vi "Run Test - Start Condition (SubVI).vi"(8 "error in (no error)":errorcluster, 9 "Time":dbl, 11 "Cluster in":T1 {"M Event" items=["Stop", "Running", "PID", "Up Limit", "Down Limit", "Load Limit"]; "Test Type" items=["Please Select", "Triaxial Shear", "Triaxial UU", "Shearbox", "Permeability", "Consolidation (Stepped Loading)/Swelling", "Saturation (Incremental)", "User Defined", "UCT", "Isotropic Consolidation", "Swelling Pressure"]; "Data"."Test Type" items=["Please Select", "Triaxial Shear", "Triaxial UU", "Shearbox", "Permeability", "Consolidation (Stepped Loading)/Swelling", "Saturation (Incremental)", "User Defined", "UCT", "Isotropic Consolidation", "Swelling Pressure"]}) -> (0 "error out":errorcluster, 2 "Delay":string, 3 "Cluster out":T1 {"M Event" items=["Stop", "Running", "PID", "Up Limit", "Down Limit", "Load Limit"]; "Test Type" items=["Please Select", "Triaxial Shear", "Triaxial UU", "Shearbox", "Permeability", "Consolidation (Stepped Loading)/Swelling", "Saturation (Incremental)", "User Defined", "UCT", "Isotropic Consolidation", "Swelling Pressure"]; "Data"."Test Type" items=["Please Select", "Triaxial Shear", "Triaxial UU", "Shearbox", "Permeability", "Consolidation (Stepped Loading)/Swelling", "Saturation (Incremental)", "User Defined", "UCT", "Isotropic Consolidation", "Swelling Pressure"]}, 5 "Enum":T10)   [LabVIEW 2019]
uses:
  Controls/RunTest - State.ctl
  Controls/RunTest - Data Structure.ctl
  Controls/Test Panel - Data Structure.ctl
  Controls/Station - Test Type.ctl
  <vilib>/Utility/miscctls.llb/LVRowAndColumnTypeDef.ctl
  Controls/RunTest - Calculate Data.ctl
  <vilib>/httpClient/ClientHandle.ctl
  Controls/RunTest - Start Condition.ctl
  Controls/RunTest - Stop Condition.ctl
  Controls/UDP - Event.ctl
  Controls/UDP - Command.ctl
  <vilib>/httpClient/LabVIEWHTTPClient.lvlib
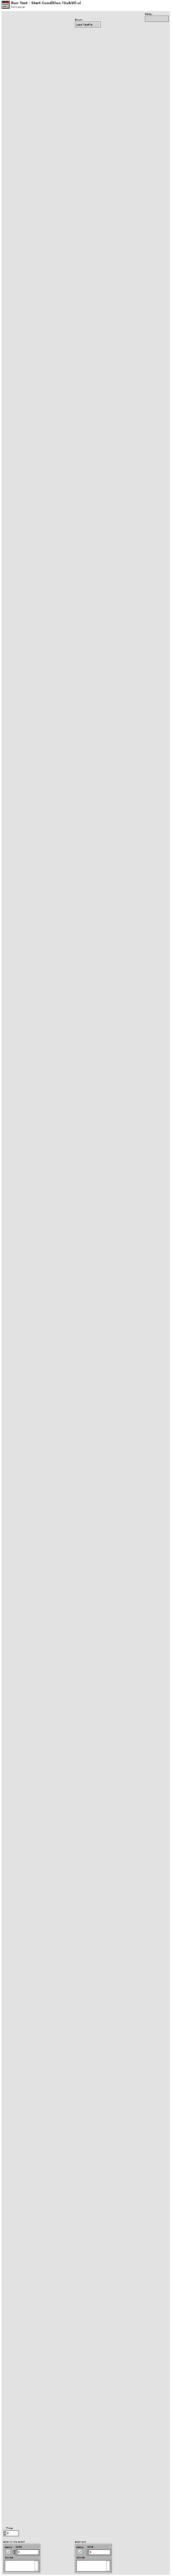
[diagram p1: front panel]
types:
  T1 = typedef "RunTest - Data Structure.ctl" = cluster{"Test Plan":string[], "PlanRow":i32, "Device Name":string[], "Timeout":i32, "Start?":bool, "Pause?":bool, "IP Address":string[], "LogRow":i32, "Logtype":u16, "Log Elapse":sgl, "Data":T2, "Stop log?":bool, "tdms":refnum<k34>, "Sensor Data":sgl[], "Start time":timestamp, "Prev Log Elapse":u32, "Plot":u16, "X-Axis":u16[], "Y-Axis":u16[], "XY":cluster{"X":dbl, "Y":dbl}[][], "End Stage?":bool, "1run":bool, "Condition":u16[], "Start Con":bool, "Log Con":bool, "Stop Con":bool, "Start Elapse":dbl, "Start Load":dbl, "Motor":i32, "StartRow":i32, "number log":i32, "Dir":bool, "Start time test":timestamp, "Auto":bool, "Check return?":bool, "Inv":cluster{"M":i32[], "Bool":bool[]}, "tdms temp":refnum<k34>, "Zero?":bool, "Plot Timer":dbl, "1st Run":bool, "TDMS Path":path, "MaxLoad":dbl, "Log Timer":sgl[], "Test Type":T3, "Log Sensor":string[], "Save?":bool, "1st Log":bool, "Y-Axis 2":u16[], "On Y-Axis 2":bool, "Decimal":u8[], "Init":cluster{"PWP TS":sgl, "Load TS":sgl, "Volume TS":sgl, "Disp TS":sgl, "CP":sgl, "Vol In":sgl, "Vol Out":sgl, "Load UCT":sgl, "Disp UCT":sgl, "PWP Sat":sgl, "CP Sat":sgl, "Volume IsoCons":sgl, "PWP IsoCons":sgl, "PWP TUU":sgl, "Load TUU":sgl, "Volume TUU":sgl, "Disp TUU":sgl, "Load Cons":sgl, "Disp Cons":sgl, "Volume Sat":sgl, "Vertical Load SB":sgl, "Vertical Disp SB":sgl, "H Disp SB":sgl, "H Load SB":sgl}, "Calc":T5, "Device Index":i32[], "Channel Index":i32[], "http ref":T6, "fileid":string, "Step Cons":cluster{"V Stress":sgl, "H Settlement":sgl}, "RunTest":bool, "Graph Last":i32, "Init?":bool, "Datalog":bool[], "Start":T7, "Stop":T8, "Running?":bool, "StartTime":dbl, "Log Prev Time":dbl, "KeyName":string[], "Test RunTime":dbl, "Log Prev Axial":dbl, "M Event":T9[], "Last Log":bool, "popup":bool, "PreStart UU":bool, "PreStart Sat":bool}
  T2 = typedef "Test Panel - Data Structure.ctl" = cluster{"Station":string, "Sample ID":string, "Job No":string, "Job Description":string, "Filename":string, "Test Type":T3, "Speciment No":string, "Depth":string, "Height":string, "Diameter/Length":string, "Weight":string, "Test Parameter":string, "Station[]":string[], "Edit Pos":T4, "Edit Pos Prev":T4, "Area":string, "Path":string}
  T3 = typedef "Station - Test Type.ctl" = u16
  T4 = typedef "LVRowAndColumnTypeDef.ctl" = cluster{"Row":i32, "Column":i32}
  T5 = typedef "RunTest - Calculate Data.ctl" = cluster{"TS":cluster{"Change PWP":sgl, "Change Vol":sgl, "Axial Load":sgl, "CiL":sgl, "Deviator":sgl, "Axial Strain":sgl, "MaxDeviator":sgl}, "TUU":cluster{"Change PWP":sgl, "Axial Load":sgl, "CiL":sgl, "Deviator":sgl, "Axial Strain":sgl, "MaxDeviator":sgl}, "Sat":cluster{"B Value":sgl, "PWP Diss":sgl, "CPP":sgl, "CV":sgl}, "Per":cluster{"Change Vol In":sgl, "Change Vol Out":sgl, "Mean Vol":sgl, "Gradient Pressure":sgl, "Outlet Flow":sgl, "Inlet Flow":sgl, "I X1":sgl, "I X2":sgl, "I Y1":sgl, "I Y2":sgl, "O X1":sgl, "O X2":sgl, "O Y1":sgl, "O Y2":sgl}, "Step Cons":cluster{"V Stress":sgl, "H Settlement":sgl, "Total H Settle":sgl, "Prev Total H":sgl}, "UCT":cluster{"ALC":sgl, "H Change":sgl, "Deviator":sgl, "Axial Strain":sgl, "V Stress":sgl, "MaxDeviator":sgl}, "ISO Cons":cluster{"CPP":sgl, "PWP Diss":sgl, "CV":sgl}, "SB":cluster{"Speci LenC":sgl, "Shear Strain":sgl, "H LC":sgl, "Normal Stress":sgl, "Shear Stress":sgl, "MaxShear":sgl}}
  T6 = typedef "LabVIEWHTTPClient.lvlib/ClientHandle.ctl" = refnum<k1>
  T7 = typedef "RunTest - Start Condition.ctl" = cluster{"Cons":cluster{"VS":dbl, "Delay":bool, "No Delay":dbl}, "Sat":cluster{"CP":dbl, "BP":dbl, "StartBP":bool, "Target CP":bool, "Target BP":bool}, "Iso":cluster{"BP":dbl}, "TS":cluster{"SS":dbl, "Engage":bool, "ES":dbl, "LC":dbl, "PreStart":bool, "Trig SS":bool, "Drain":dbl}, "TUU":cluster{"SS":dbl, "Engage":bool, "ES":dbl, "LC":dbl, "PreStart":bool, "Trig SS":bool, "CP":dbl, "Delay Value":dbl, "Delay":bool, "CP PID":bool}, "UCT":cluster{"SS":dbl, "Engage":bool, "ES":dbl, "LC":dbl, "PreStart":bool, "Trig SS":bool}, "Enable?":bool, "SB":cluster{"SS":dbl, "Engage":bool, "ES":dbl, "LC":dbl, "PreStart":bool, "Trig SS":bool, "VS":dbl, "Delay Value":dbl, "Delay":bool, "VS PID":bool}, "Perm":cluster{"DP":dbl}}
  T8 = typedef "RunTest - Stop Condition.ctl" = cluster{"Cons":cluster{"Select":i32, "Disp":dbl, "Time":dbl, "Time2":dbl, "Disp 2":dbl, "Time Cond":dbl, "Last Disp":dbl, "Swell":bool}, "Sat":cluster{"Select":i32, "PP":dbl, "Time":dbl, "VC":dbl, "Time2":dbl, "Time Cond":dbl, "Last PP":dbl, ".B":bool, "B":dbl, "Last Vc":dbl, "Time Cond 2":dbl, "Time3":dbl, "Time Cond 3":dbl}, "Iso":cluster{"PP":dbl, "Time":dbl, "VC":dbl, "Time2":dbl, "Time Cond":dbl, "Last Vc":dbl, ".PP":bool, "Time Cond 2":dbl, "Select":i32}, "TS":cluster{"Axial":dbl, ".MaxDev":bool, "MaxDev Value":dbl, "Return":bool, "Reset":bool, "Prev Time":dbl, "PostStop Run":bool, "CP Stop":bool, "BP Stop":bool, "PostStop Trig":bool, "Reset Value":dbl, "BPTrig":bool, "CPTrig":bool, "VLCTrig":bool}, "TUU":cluster{"Axial":dbl, ".MaxDev":bool, "MaxDev Value":dbl, "Return":bool, "Reset":bool, "Prev Time":dbl, "PostStop Run":bool, "CP Stop":bool, "BP Stop":bool, "PostStop Trig":bool, "Reset Value":dbl, "BPTrig":bool, "CPTrig":bool, "VLCTrig":bool}, "UCT":cluster{"Axial":dbl, ".MaxDev":bool, "MaxDev Value":dbl, "Return":bool, "Reset":bool, "Prev Time":dbl, "PostStop Run":bool, "CP Stop":bool, "BP Stop":bool, "PostStop Trig":bool}, "Enable?":bool, "SB":cluster{"Shear":dbl, ".MaxShear":bool, "MaxShear Value":dbl, "Return":bool, "Reset":bool, "Prev Time":dbl, "PostStop Run":bool, "CP Stop":bool, "BP Stop":bool, "PostStop Trig":bool, "Reset Value":dbl, "BPTrig":bool, "CPTrig":bool, "VLCTrig":bool}, "Perm":cluster{"Max Time":bool, "Reset":bool, "PostStop Run":bool, "Ratio":bool, "Reset Value":dbl, "Time":dbl, "RatioTime":dbl, "RatioMore":dbl, "RatioLess":dbl, "Time Cond":dbl, "Time Cond 2":dbl, "Prev IF":dbl, "Prev OF":dbl, "PostStop Trig":bool, "BP Trig":bool, "DP Stop":bool, "BP Stop":bool, "CP Stop":bool, "CP Trig":bool}, "SP":cluster{".Max Time":bool, ".Time":bool, "Time":dbl, "MaxTime":dbl, "Time Cond":dbl, "Max Time Cond":dbl, "Stress":dbl}}
  T9 = typedef "UDP - Event.ctl" = u16
  T10 = typedef "RunTest - State.ctl" = enum16{"Load Testfile", "Notifier", "Init", "Idle", "Load", "Read DB", "Run", "Pause", "Stop", "Check Start", "Check Stop", "Check Post Stop", "Check Log", "EndStage", "Data View", "Display", "Graph", "Graph Old", "Close", "Stop PID", "Check Limit", "Auto", "Up", "Log", "Zero", "Machine Control", "Save Report"}
  T11 = enum32{"Please Select", "Triaxial Shear", "Triaxial UU", "Shearbox", "Permeability", "Consolidation", "Saturation", "User Defined", "UCT", "Iso Consolidation"}
  T12 = cluster{"Target Load":sgl, "Target Disp":sgl, "Rate":sgl, "Speed":sgl}
  T13 = enum16{"None", "Run Target", "Run Ramp", "Run Disp"}
  T14 = typedef "UDP - Command.ctl" = enum16{"Stop", "Jog Up", "Jog Down", "Ramp Up", "Ramp Down", "PID Target", "PID Ramp", "Disp Run", "Read Ch Data", "Zero Channel", "Zero Disp", "Read Sensor", "Write Sensor", "Read ADC", "Write ADC", "Read PID", "Write PID", "Read Test", "Write Test", "Read System", "Write System", "Read Datalog", "Read Datalog Sensor"}
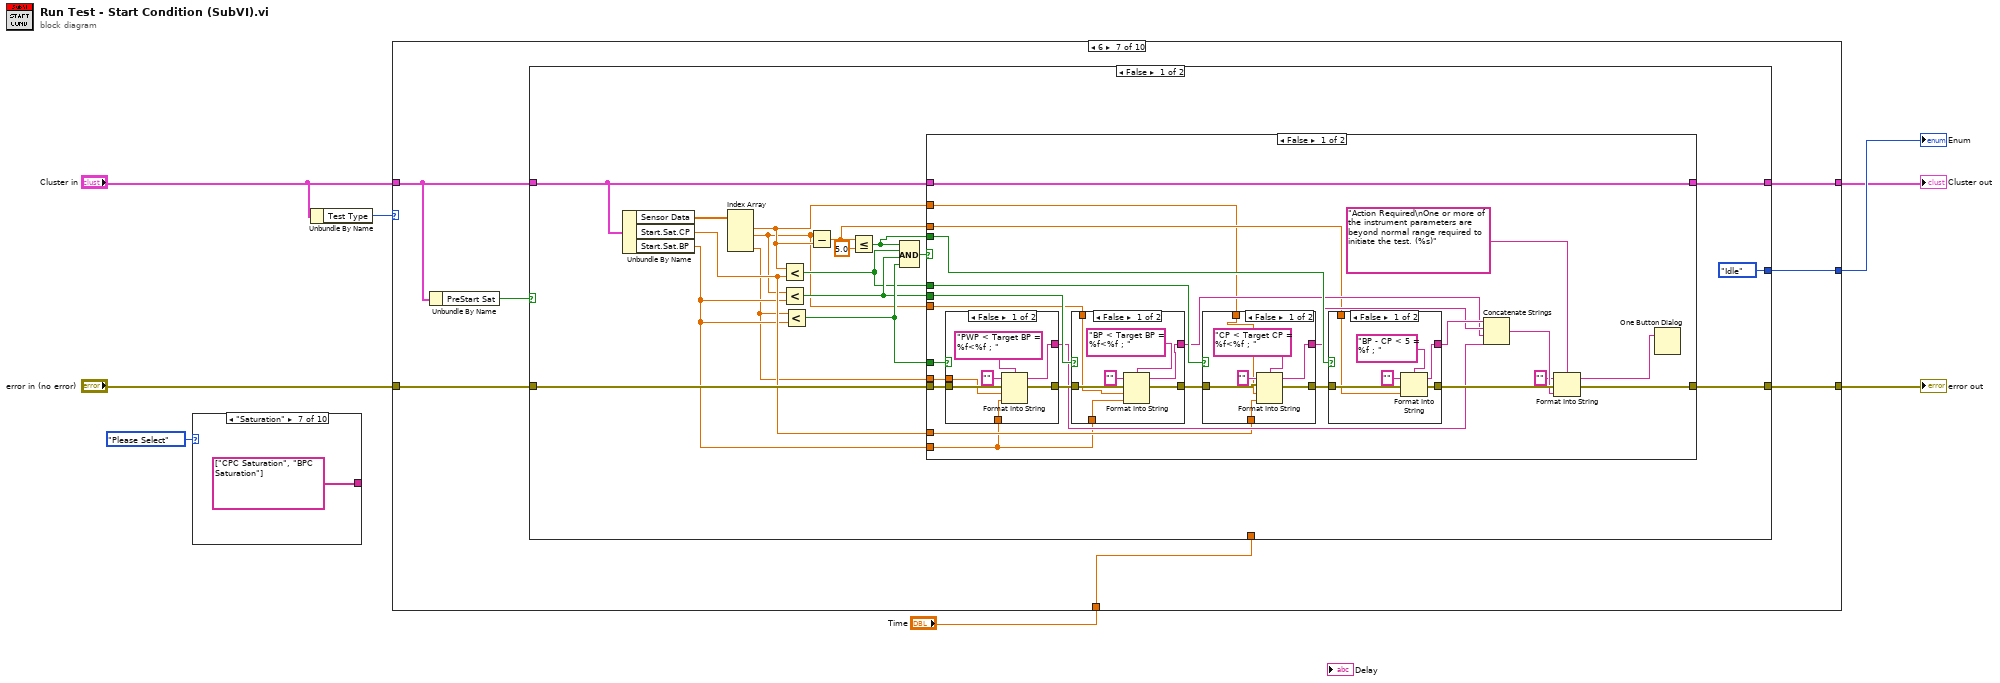
[diagram p0: block diagram]
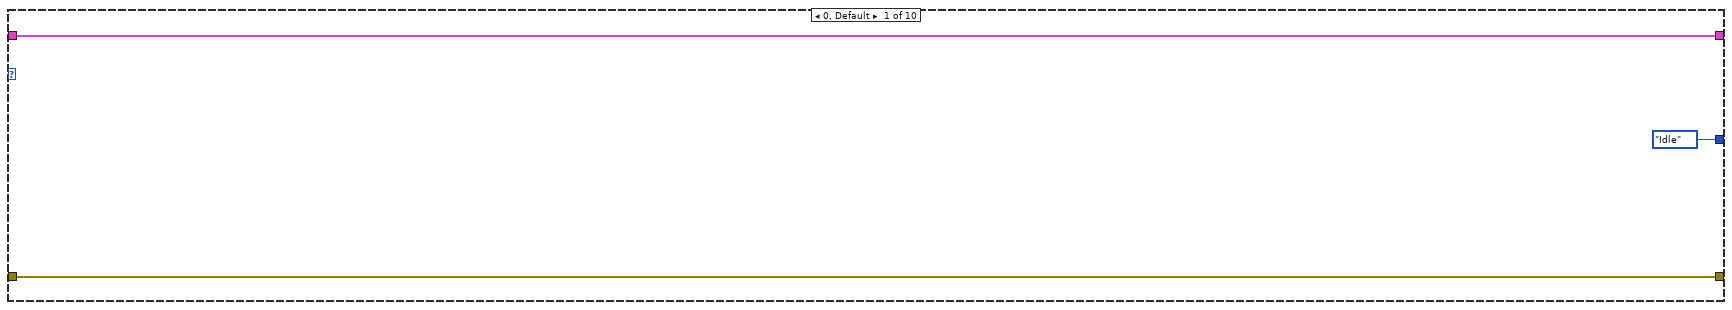
[diagram p2: hidden frame]
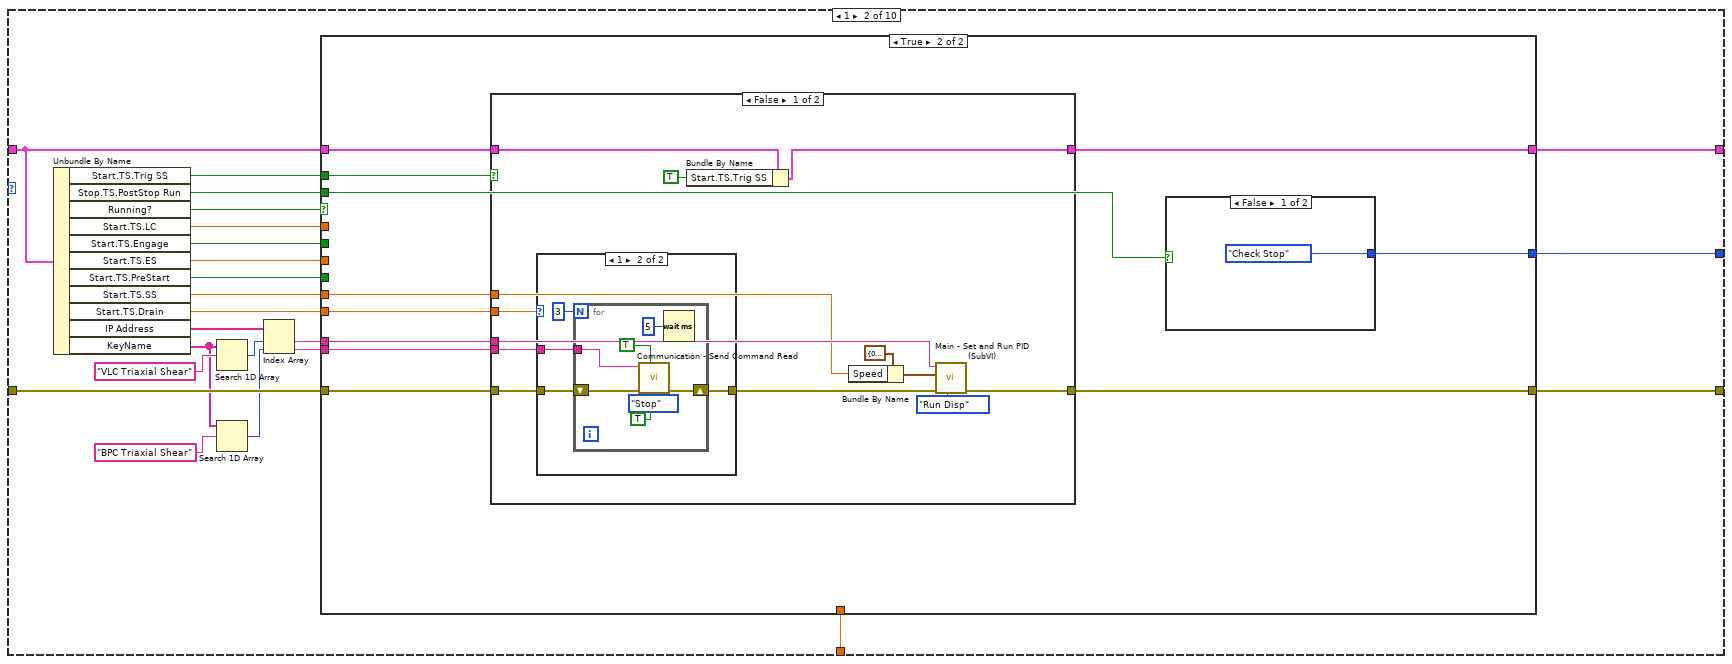
[diagram p3: hidden frame]
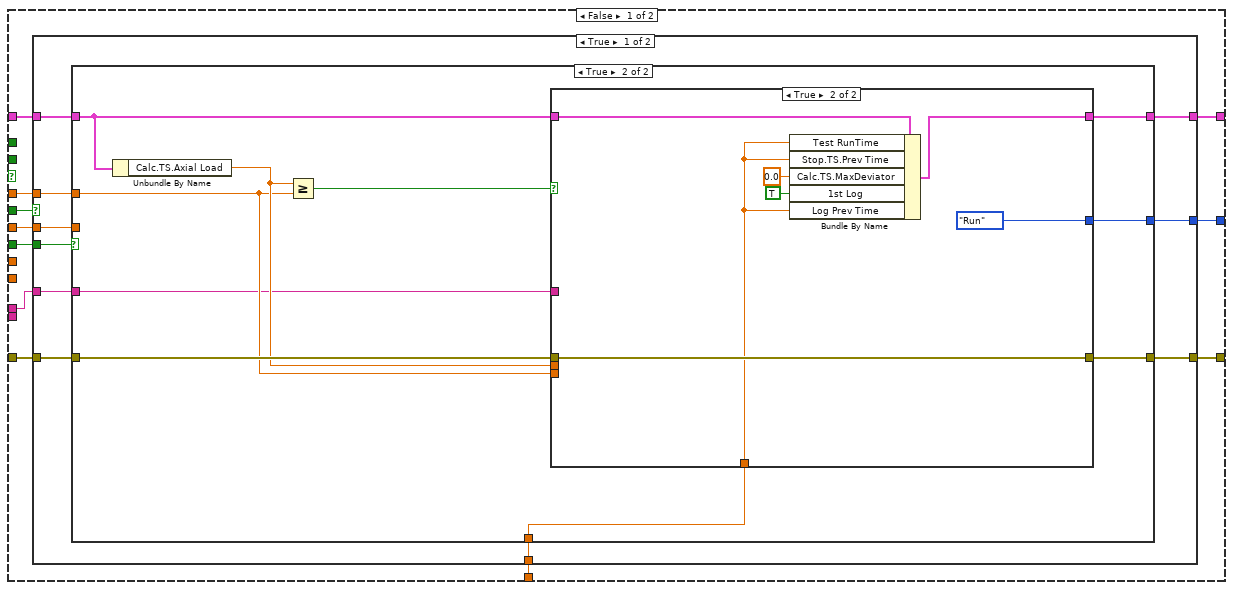
[diagram p4: hidden frame]
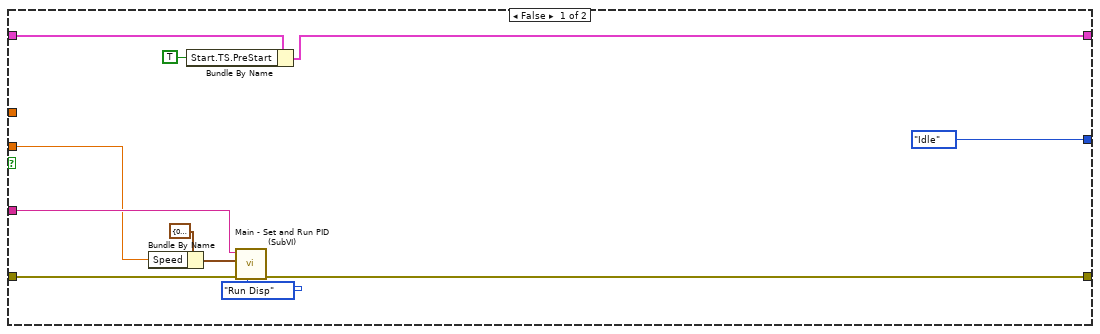
[diagram p5: hidden frame]
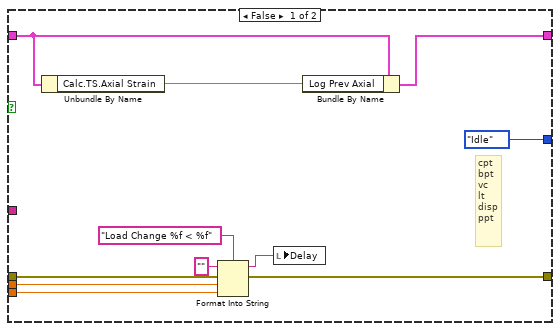
[diagram p6: hidden frame]
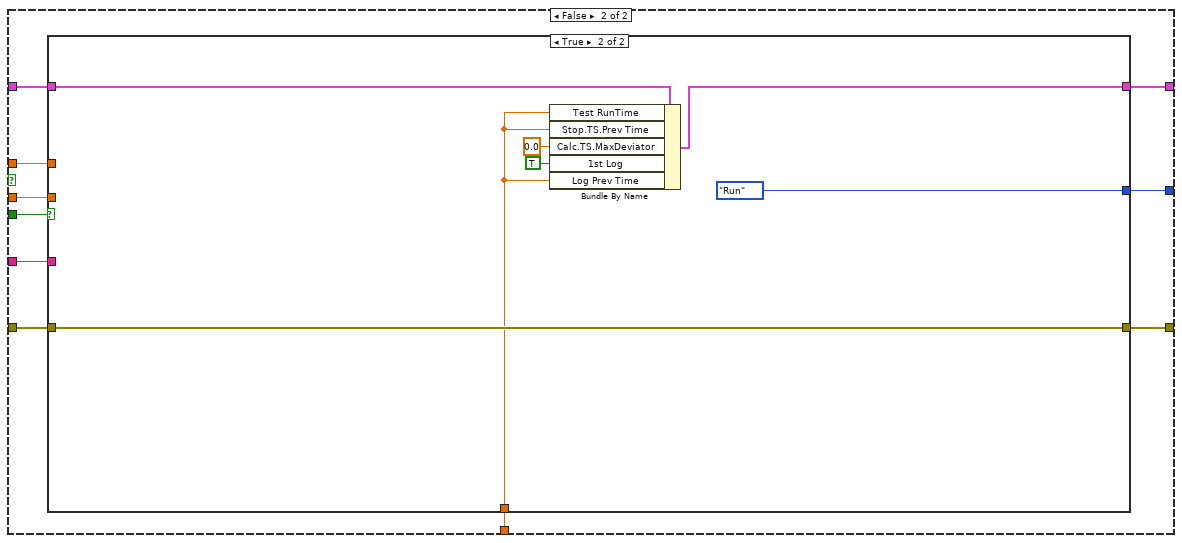
[diagram p7: hidden frame]
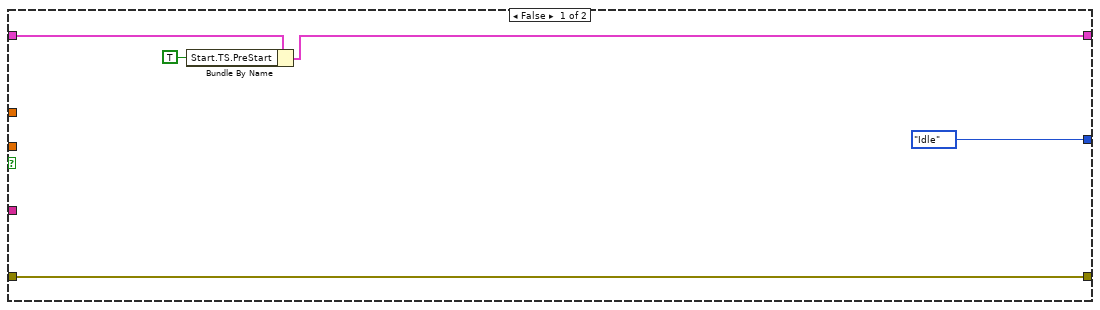
[diagram p8: hidden frame]
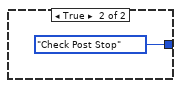
[diagram p11: hidden frame]
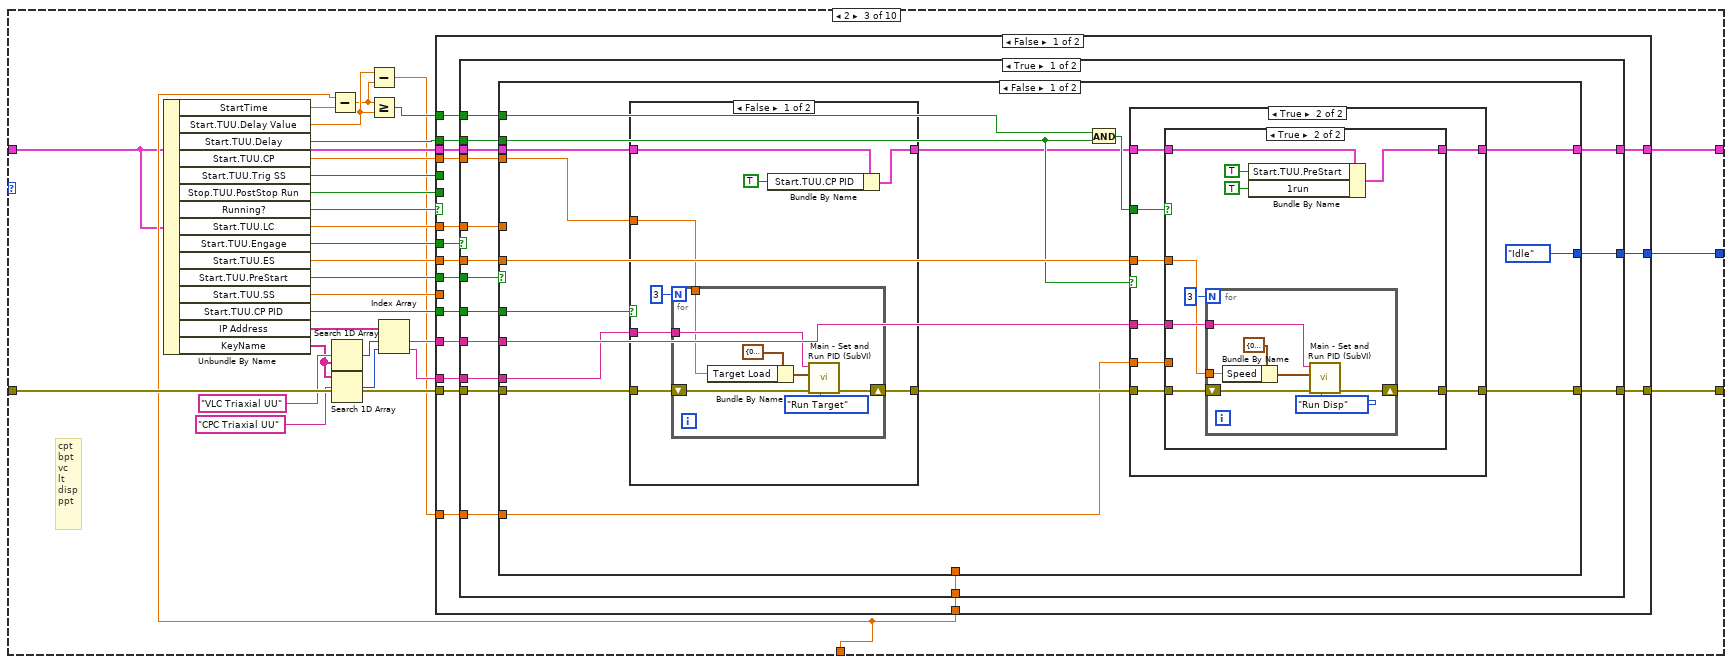
[diagram p12: hidden frame]
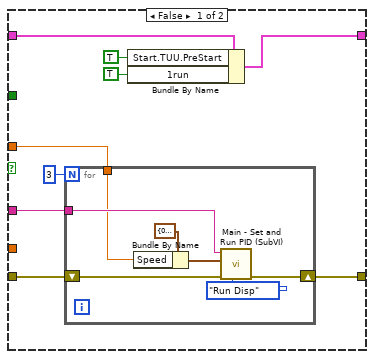
[diagram p13: hidden frame]
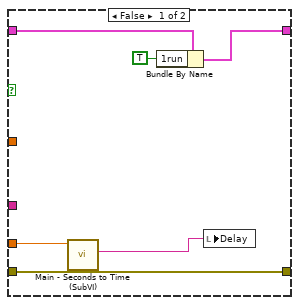
[diagram p14: hidden frame]
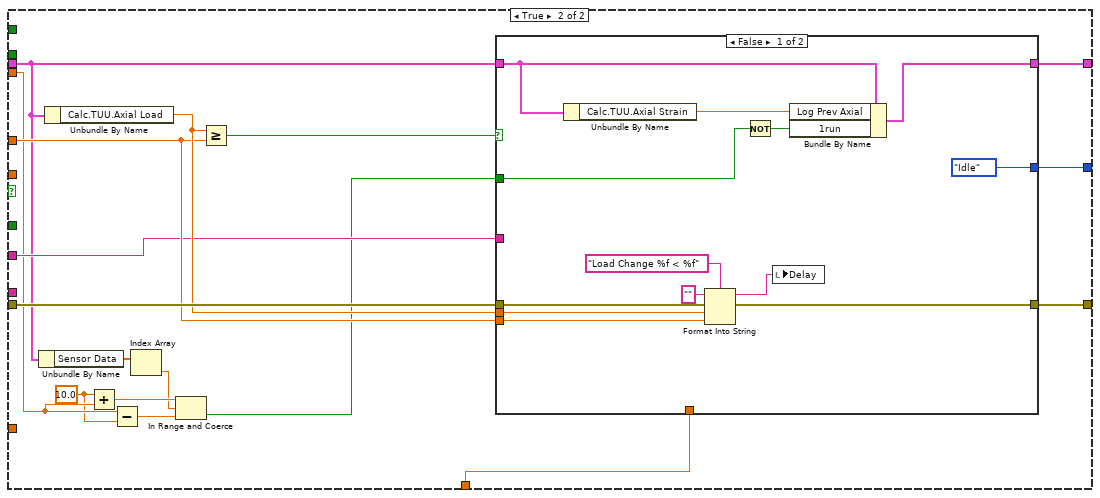
[diagram p16: hidden frame]
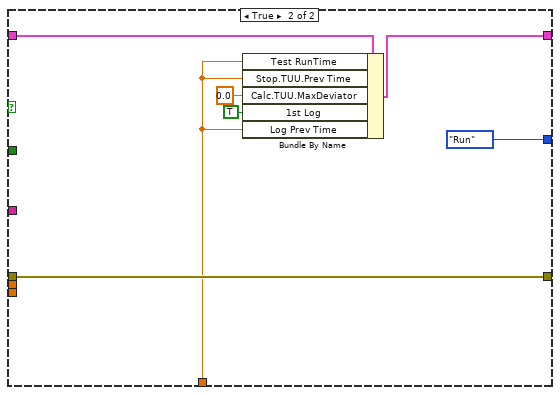
[diagram p17: hidden frame]
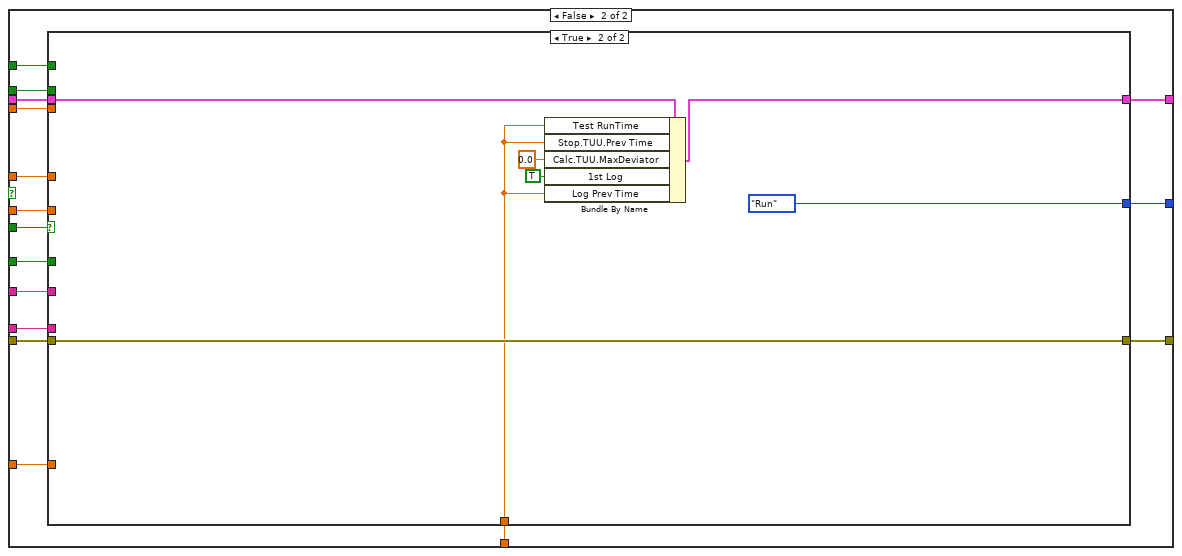
[diagram p18: hidden frame]
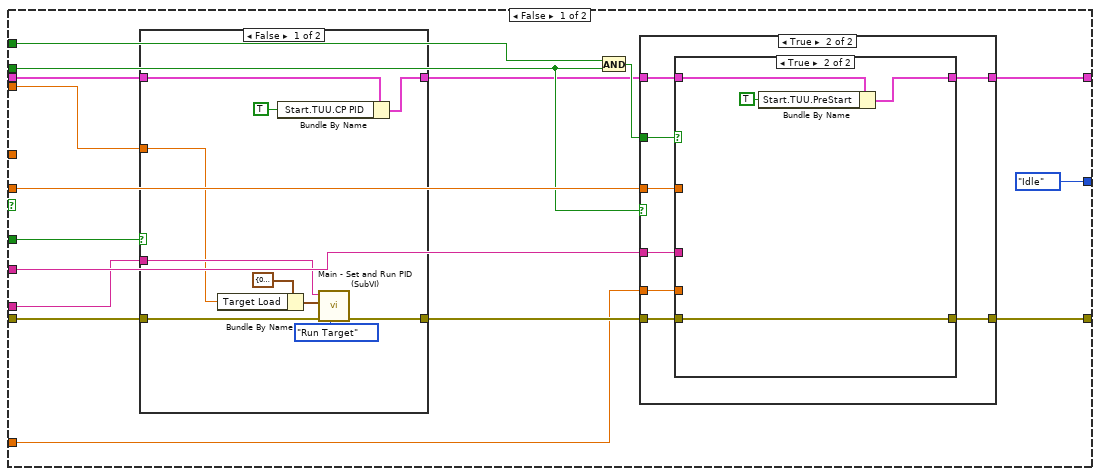
[diagram p19: hidden frame]
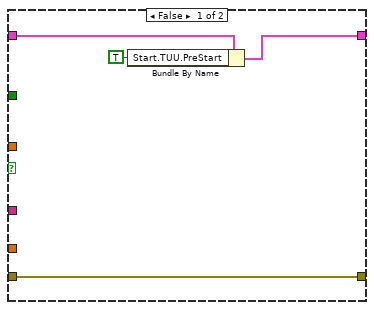
[diagram p20: hidden frame]
diagram:
  n1 = case shown="\"Saturation\"" T11."Please Select" ("Sub Tab") {
    tunnel: [string[] [] string[] ["CPC Triaxial Shear", "BPC Triaxial Shear", "VLC Triaxial Shear"] string[] ["CPC Triaxial UU", "VLC Triaxial UU"] string[] ["VLC Shearbox", "HLC Shearbox"] string[] ["CPC Permeability", "BPC Permeability", "BPC2 Permeability"] string[] ["VLC Consolidation"] string[] ["CPC Saturation", "BPC Saturation"] string[] ["CPC User Defined", "BPC User Defined", "BPC2 User Defined", "VLC User Defined", "HLC User Defined"] string[] ["VLC UCT"] string[] ["CPC Iso", "BPC Iso"]] -> _
    frame "Please Select", Default {
    }
    frame "Triaxial Shear" {
    }
    frame "Triaxial UU" {
    }
    frame "Shearbox" {
    }
    frame "Permeability" {
    }
    frame "Consolidation" {
    }
    frame "Saturation" {
    }
    frame "User Defined" {
    }
    frame "UCT" {
    }
    frame "Iso Consolidation" {
    }
  }
  n2 = Unbundle By Name("Cluster in") -> ("Test Type"=w1:T3)
  n3 = case shown="6" w1 {
    tunnel: [w21 w39 w195 w464 w708 w773 w953 w1243 w1359 w1426] -> w3
    tunnel: "Cluster in" -> [w21 w40 w191 w465 w707 w772 w951 w1244 w1358 w1425]
    tunnel: [w20 w38 w194 w463 w714 w779 w956 w1242 w1364 w1430] -> w5
    tunnel: "error in (no error)" -> [w20 w43 w196 w468 w713 w778 w955 w1247 w1363 w1429]
    tunnel: [RunTest_-_State."Idle" w36 w193 w461 w712 w777 w954 w1240 w1362 w1428] -> w6
    tunnel: "Time" -> [_ w27 w192 w440 w702 w765 w952 w1230 w1354 w1424]
    frame 0, Default {
    }
    frame 1 {
      n4 = Unbundle By Name(w40) -> ("Start.TS.Trig SS"=w28:bool, "Stop.TS.PostStop Run"=w29:bool, "Running?"=w31:bool, "Start.TS.LC"=w37:dbl, "Start.TS.Engage"=w41:bool, "Start.TS.ES"=w42:dbl, "Start.TS.PreStart"=w44:bool, "Start.TS.SS"=w30:dbl, "Start.TS.Drain"=w22:dbl, "IP Address"=w34:string[], "KeyName"=w25:string[])
      n5 = Search 1D Array(1D array=w25, element="VLC Triaxial Shear" ("String")) -> (index of element=w35:i32)  [unwired: 1 in]
      n6 = Search 1D Array(1D array=w25, element="BPC Triaxial Shear" ("String")) -> (index of element=w24:i32)  [unwired: 1 in]
      n7 = Index Array(array=w34, index #1=w35, index #2=w24) -> (element #1=w32:string, element #2=w23:string)
      n8 = case shown="True" w31 {
        tunnel: w44 -> [w55 _]
        tunnel: w43 -> [w54 w134]
        tunnel: w42 -> [w53 _]
        tunnel: w41 -> [w52 _]
        tunnel: w40 -> [w51 w129]
        tunnel: [w50 w130] -> w39
        tunnel: [w49 w135] -> w38
        tunnel: w37 -> [w48 _]
        tunnel: [w47 w137] -> w36
        tunnel: w32 -> [w46 w133]
        tunnel: w30 -> [_ w132]
        tunnel: w29 -> [_ w136]
        tunnel: w28 -> [_ w131]
        tunnel: w27 -> [w45 _]
        tunnel: w23 -> [_ w128]
        tunnel: w22 -> [_ w127]
        frame False {
          n9 = case shown="True" w52 {
            tunnel: w55 -> [w65 w114]
            tunnel: w54 -> [w64 w113]
            tunnel: w53 -> [w63 w112]
            tunnel: [w62 w111] -> w49
            tunnel: w51 -> [w61 w110]
            tunnel: [w60 w109] -> w50
            tunnel: w48 -> [w59 w108]
            tunnel: [w58 w107] -> w47
            tunnel: w46 -> [w57 w106]
            tunnel: w45 -> [w56 w105]
            frame True {
              n10 = case shown="True" w65 {
                tunnel: w64 -> [w73 w84]
                tunnel: [w72 w85] -> w62
                tunnel: w63 -> [w66 _]
                tunnel: w61 -> [w71 w78]
                tunnel: [w69 w79] -> w60
                tunnel: w59 -> [_ w82]
                tunnel: [RunTest_-_State."Idle" w86] -> w58
                tunnel: w57 -> [w68 w80]
                tunnel: w56 -> [_ w77]
                frame False {
                  n11 = Bundle By Name(cluster=T12 {"Target Load"=0.0, "Target Disp"=0.0, "Rate"=0.0, "Speed"=0.0} ("Test"), "Speed"=w66) -> (w76:T12)
                  n12 = Bundle By Name(cluster=w71, "Start.TS.PreStart"=TRUE) -> (w69:T1)
                  n13 = call "Main - Set and Run PID (SubVI).vi"("Action"=T13."Run Disp", "error in (no error)"=w73, "Test"=w76, "IP Address"=w68) -> ("error out"=w72:errorcluster)  [unwired: 7 in]
                }
                frame True {
                  n14 = Unbundle By Name(w78) -> ("Calc.TS.Axial Load"=w83:sgl)
                  n15 = Greater Or Equal?(x=w83, y=w82) -> (x >= y?=w81:bool)
                  n16 = case shown="True" w81 {
                    tunnel: [RunTest_-_State."Idle" RunTest_-_State."Run"] -> w86
                    tunnel: [w97 w100] -> w85
                    tunnel: w84 -> [w96 w100]
                    tunnel: w83 -> [w94 _]
                    tunnel: w82 -> [w93 _]
                    tunnel: w80 -> [_ _]
                    tunnel: [w90 w103] -> w79
                    tunnel: w78 -> [w89 w102]
                    tunnel: w77 -> [_ w98]
                    frame False {
                      # "cpt\nbpt\nvc\nlt\ndisp\nppt"
                      n17 = Unbundle By Name(w89) -> ("Calc.TS.Axial Strain"=w88:sgl)
                      n18 = Format Into String(format string="Load Change %f < %f" ("Delay"), initial string="", error in=w96, w94, w93) -> (resulting string=w87:string, error out=w97:errorcluster)
                      n19 = local write "Delay"(w87) -> ()
                      n20 = Bundle By Name(cluster=w89, "Log Prev Axial"=w88) -> (w90:T1)
                    }
                    frame True {
                      n21 = Bundle By Name(cluster=w102, "Test RunTime"=w98, "Stop.TS.Prev Time"=w98, "Calc.TS.MaxDeviator"=sgl 0.0, "1st Log"=TRUE, "Log Prev Time"=w98) -> (w103:T1)
                    }
                  }
                }
              }
            }
            frame False {
              n22 = case shown="True" w114 {
                tunnel: w113 -> [w119 w125]
                tunnel: [w119 w125] -> w111
                tunnel: w112 -> [_ _]
                tunnel: w110 -> [w118 w123]
                tunnel: [w116 w124] -> w109
                tunnel: w108 -> [_ _]
                tunnel: [RunTest_-_State."Idle" RunTest_-_State."Run"] -> w107
                tunnel: w106 -> [_ _]
                tunnel: w105 -> [_ w122]
                frame False {
                  n23 = Bundle By Name(cluster=w118, "Start.TS.PreStart"=TRUE) -> (w116:T1)
                }
                frame True {
                  n24 = Bundle By Name(cluster=w123, "Test RunTime"=w122, "Stop.TS.Prev Time"=w122, "Calc.TS.MaxDeviator"=sgl 0.0, "1st Log"=TRUE, "Log Prev Time"=w122) -> (w124:T1)
                }
              }
            }
          }
        }
        frame True {
          n25 = case shown="False" w131 {
            tunnel: [w148 w163] -> w135
            tunnel: w134 -> [w141 w163]
            tunnel: w133 -> [w147 _]
            tunnel: w132 -> [w143 _]
            tunnel: [w146 w164] -> w130
            tunnel: w129 -> [w145 w164]
            tunnel: w128 -> [w140 _]
            tunnel: w127 -> [w142 _]
            frame False {
              n26 = case shown="1" w142 {
                tunnel: w141 -> [w151 w155]
                tunnel: w140 -> [_ w153]
                tunnel: [w151 w154] -> w139
                frame 0, Default {
                }
                frame 1 {
                  n27 = for {
                    N: 3 -> [_]
                    tunnel: w153 -> [w157]
                    shift-right: [w158] -> w154
                    shift-left: w155 -> [w159]
                    n28 = call "Communication - Send Command Read.vi"("Fron?"=TRUE, "Bypass?"=TRUE, "error in (no error)"=w159, "Action"=UDP_-_Command."Stop", "Device IP Address"=w157) -> ("error out"=w158:errorcluster)  [unwired: 6 in]
                    n29 = Wait (ms)(milliseconds to wait=u32 5) -> ()  [unwired: 1 out]
                  }
                }
              }
              n30 = Bundle By Name(cluster=w145, "Start.TS.Trig SS"=TRUE) -> (w146:T1)
              n31 = Bundle By Name(cluster=T12 {"Target Load"=0.0, "Target Disp"=0.0, "Rate"=0.0, "Speed"=0.0} ("Test"), "Speed"=w143) -> (w150:T12)
              n32 = call "Main - Set and Run PID (SubVI).vi"("Action"=T13."Run Disp", "error in (no error)"=w139, "Test"=w150, "IP Address"=w147) -> ("error out"=w148:errorcluster)  [unwired: 7 in]
            }
            frame True {
            }
          }
          n33 = case shown="False" w136 {
            tunnel: [RunTest_-_State."Check Stop" RunTest_-_State."Check Post Stop"] -> w137
            frame False {
            }
            frame True {
            }
          }
        }
      }
    }
    frame 2 {
      # "cpt\nbpt\nvc\nlt\ndisp\nppt"
      n34 = Unbundle By Name(w191) -> ("StartTime"=w172:dbl, "Start.TUU.Delay Value"=w169:dbl, "Start.TUU.Delay"=w173:bool, "Start.TUU.CP"=w178:dbl, "Start.TUU.Trig SS"=w179:bool, "Stop.TUU.PostStop Run"=w180:bool, "Running?"=w182:bool, "Start.TUU.LC"=w187:dbl, "Start.TUU.Engage"=w188:bool, "Start.TUU.ES"=w189:dbl, "Start.TUU.PreStart"=w190:bool, "Start.TUU.SS"=w181:dbl, "Start.TUU.CP PID"=w170:bool, "IP Address"=w185:string[], "KeyName"=w177:string[])
      n35 = Subtract(x=w192, y=w172) -> (x-y=w168:dbl)
      n36 = Search 1D Array(1D array=w177, element="VLC Triaxial UU" ("String")) -> (index of element=w186:i32)  [unwired: 1 in]
      n37 = Search 1D Array(1D array=w177, element="CPC Triaxial UU" ("String")) -> (index of element=w175:i32)  [unwired: 1 in]
      n38 = Subtract(x=w169, y=w168) -> (x-y=w167:dbl)
      n39 = Greater Or Equal?(x=w168, y=w169) -> (x >= y?=w171:bool)
      n40 = Index Array(array=w185, index #1=w186, index #2=w175) -> (element #1=w183:string, element #2=w174:string)
      n41 = case shown="False" w182 {
        tunnel: w190 -> [w213 _]
        tunnel: w196 -> [w212 w422]
        tunnel: w189 -> [w211 _]
        tunnel: w188 -> [w210 _]
        tunnel: w191 -> [w209 w417]
        tunnel: [w208 w418] -> w195
        tunnel: [w207 w423] -> w194
        tunnel: w187 -> [w206 _]
        tunnel: [w205 w425] -> w193
        tunnel: w183 -> [w204 w421]
        tunnel: w181 -> [_ w420]
        tunnel: w180 -> [_ w424]
        tunnel: w179 -> [_ w419]
        tunnel: w178 -> [w203 _]
        tunnel: w174 -> [w202 _]
        tunnel: w173 -> [w201 _]
        tunnel: w171 -> [w200 _]
        tunnel: w170 -> [w199 _]
        tunnel: w167 -> [w198 _]
        tunnel: w192 -> [w197 _]
        frame False {
          n42 = case shown="True" w210 {
            tunnel: w213 -> [w229 w361]
            tunnel: w212 -> [w228 w360]
            tunnel: w211 -> [w227 w359]
            tunnel: [w226 w358] -> w207
            tunnel: w209 -> [w225 w357]
            tunnel: [w224 w356] -> w208
            tunnel: w206 -> [w223 w355]
            tunnel: [w222 w354] -> w205
            tunnel: w204 -> [w221 w353]
            tunnel: w203 -> [w220 w352]
            tunnel: w202 -> [w219 w351]
            tunnel: w201 -> [w218 w350]
            tunnel: w200 -> [w217 w349]
            tunnel: w199 -> [w216 w348]
            tunnel: w198 -> [w215 w347]
            tunnel: w197 -> [w214 w346]
            frame True {
              n43 = case shown="False" w229 {
                tunnel: w228 -> [w237 w323]
                tunnel: [w239 w324] -> w226
                tunnel: w227 -> [w242 _]
                tunnel: w225 -> [w232 w313]
                tunnel: [w245 w319] -> w224
                tunnel: w223 -> [_ w321]
                tunnel: [RunTest_-_State."Idle" w325] -> w222
                tunnel: w221 -> [w244 w320]
                tunnel: w220 -> [w240 w311]
                tunnel: w219 -> [w241 _]
                tunnel: w218 -> [w235 _]
                tunnel: w217 -> [w236 _]
                tunnel: w216 -> [w233 _]
                tunnel: w215 -> [w231 _]
                tunnel: w214 -> [_ w318]
                frame False {
                  n44 = case shown="False" w233 {
                    tunnel: w241 -> [w299 _]
                    tunnel: w240 -> [w293 _]
                    tunnel: [w298 w307] -> w238
                    tunnel: w237 -> [w297 w307]
                    tunnel: [w296 w308] -> w230
                    tunnel: w232 -> [w295 w308]
                    frame False {
                      n45 = for {
                        N: 3 -> [_]
                        tunnel: w299 -> [w303]
                        tunnel: w293 -> [w300]
                        shift-right: [w302] -> w298
                        shift-left: w297 -> [w301]
                        n46 = Bundle By Name(cluster=T12 {"Target Load"=0.0, "Target Disp"=0.0, "Rate"=0.0, "Speed"=0.0} ("Test"), "Target Load"=w300) -> (w304:T12)
                        n47 = call "Main - Set and Run PID (SubVI).vi"("Action"=T13."Run Target", "error in (no error)"=w301, "Test"=w304, "IP Address"=w303) -> ("error out"=w302:errorcluster)  [unwired: 7 in]
                      }
                      n48 = Bundle By Name(cluster=w295, "Start.TUU.CP PID"=TRUE) -> (w296:T1)
                    }
                    frame True {
                    }
                  }
                  n49 = And(x=w236, y=w235) -> (x .and. y?=w234:bool)
                  n50 = case shown="True" w235 {
                    tunnel: w230 -> [w254 w269]
                    tunnel: [w253 w268] -> w245
                    tunnel: w244 -> [w252 w267]
                    tunnel: w242 -> [w251 w266]
                    tunnel: [w250 w265] -> w239
                    tunnel: w238 -> [w249 w264]
                    tunnel: w234 -> [_ w263]
                    tunnel: w231 -> [_ w262]
                    frame False {
                      n51 = for {
                        N: 3 -> [_]
                        tunnel: w252 -> [w258]
                        tunnel: w251 -> [w257]
                        shift-right: [w256] -> w250
                        shift-left: w249 -> [w255]
                        n52 = Bundle By Name(cluster=T12 {"Target Load"=0.0, "Target Disp"=0.0, "Rate"=0.0, "Speed"=0.0} ("Test"), "Speed"=w257) -> (w261:T12)
                        n53 = call "Main - Set and Run PID (SubVI).vi"("Action"=T13."Run Disp", "error in (no error)"=w255, "Test"=w261, "IP Address"=w258) -> ("error out"=w256:errorcluster)  [unwired: 7 in]
                      }
                      n54 = Bundle By Name(cluster=w254, "Start.TUU.PreStart"=TRUE, "1run"=TRUE) -> (w253:T1)
                    }
                    frame True {
                      n55 = case shown="True" w263 {
                        tunnel: w269 -> [w270 w284]
                        tunnel: [w271 w283] -> w268
                        tunnel: w267 -> [_ w282]
                        tunnel: w266 -> [_ w281]
                        tunnel: [w275 w280] -> w265
                        tunnel: w264 -> [w275 w279]
                        tunnel: w262 -> [w274 _]
                        frame False {
                          n56 = call "Main - Seconds to Time (SubVI).vi"("Seconds"=w274) -> ("Time string"=w273:string)  [unwired: 9 in, 1 out]
                          n57 = Bundle By Name(cluster=w270, "1run"=TRUE) -> (w271:T1)
                          n58 = local write "Delay"(w273) -> ()
                        }
                        frame True {
                          n59 = for {
                            N: 3 -> [_]
                            tunnel: w282 -> [w288]
                            tunnel: w281 -> [w287]
                            shift-right: [w286] -> w280
                            shift-left: w279 -> [w285]
                            n60 = Bundle By Name(cluster=T12 {"Target Load"=0.0, "Target Disp"=0.0, "Rate"=0.0, "Speed"=0.0} ("Test"), "Speed"=w287) -> (w291:T12)
                            n61 = call "Main - Set and Run PID (SubVI).vi"("Action"=T13."Run Disp", "error in (no error)"=w285, "Test"=w291, "IP Address"=w288) -> ("error out"=w286:errorcluster)  [unwired: 7 in]
                          }
                          n62 = Bundle By Name(cluster=w284, "Start.TUU.PreStart"=TRUE, "1run"=TRUE) -> (w283:T1)
                        }
                      }
                    }
                  }
                }
                frame True {
                  w310 = 10.0 ("x")
                  n63 = Unbundle By Name(w313) -> ("Sensor Data"=w315:sgl[])
                  n64 = Unbundle By Name(w313) -> ("Calc.TUU.Axial Load"=w322:sgl)
                  n65 = Add(x=w310, y=w311) -> (x+y=w317:dbl)
                  n66 = Subtract(x=w311, y=w310) -> (x-y=w316:dbl)
                  n67 = Index Array(array=w315) -> (element=w314:sgl)  [unwired: 1 in]
                  n68 = In Range and Coerce(upper limit=w317, x=w314, lower limit=w316) -> (In Range?=w309:bool)  [unwired: 1 out]
                  n69 = Greater Or Equal?(x=w322, y=w321) -> (x >= y?=w312:bool)
                  n70 = case shown="False" w312 {
                    tunnel: [RunTest_-_State."Idle" RunTest_-_State."Run"] -> w325
                    tunnel: [w338 w341] -> w324
                    tunnel: w323 -> [w337 w341]
                    tunnel: w322 -> [w335 _]
                    tunnel: w321 -> [w334 _]
                    tunnel: w320 -> [_ _]
                    tunnel: [w331 w344] -> w319
                    tunnel: w313 -> [w330 w343]
                    tunnel: w318 -> [_ w339]
                    tunnel: w309 -> [w327 _]
                    frame False {
                      n71 = Unbundle By Name(w330) -> ("Calc.TUU.Axial Strain"=w329:sgl)
                      n72 = Format Into String(format string="Load Change %f < %f" ("Delay"), initial string="", error in=w337, w335, w334) -> (resulting string=w328:string, error out=w338:errorcluster)
                      n73 = Not(x=w327) -> (.not. x?=w326:bool)
                      n74 = local write "Delay"(w328) -> ()
                      n75 = Bundle By Name(cluster=w330, "Log Prev Axial"=w329, "1run"=w326) -> (w331:T1)
                    }
                    frame True {
                      n76 = Bundle By Name(cluster=w343, "Test RunTime"=w339, "Stop.TUU.Prev Time"=w339, "Calc.TUU.MaxDeviator"=sgl 0.0, "1st Log"=TRUE, "Log Prev Time"=w339) -> (w344:T1)
                    }
                  }
                }
              }
            }
            frame False {
              n77 = case shown="True" w361 {
                tunnel: w360 -> [w369 w415]
                tunnel: [w371 w415] -> w358
                tunnel: w359 -> [w374 _]
                tunnel: w357 -> [w363 w413]
                tunnel: [w377 w414] -> w356
                tunnel: w355 -> [_ _]
                tunnel: [RunTest_-_State."Idle" RunTest_-_State."Run"] -> w354
                tunnel: w353 -> [w376 _]
                tunnel: w352 -> [w372 _]
                tunnel: w351 -> [w373 _]
                tunnel: w350 -> [w367 _]
                tunnel: w349 -> [w368 _]
                tunnel: w348 -> [w365 _]
                tunnel: w347 -> [w362 _]
                tunnel: w346 -> [_ w412]
                frame False {
                  n78 = case shown="False" w365 {
                    tunnel: w373 -> [w404 _]
                    tunnel: w372 -> [w403 _]
                    tunnel: [w402 w408] -> w370
                    tunnel: w369 -> [w401 w408]
                    tunnel: [w400 w409] -> w364
                    tunnel: w363 -> [w399 w409]
                    frame False {
                      n79 = Bundle By Name(cluster=T12 {"Target Load"=0.0, "Target Disp"=0.0, "Rate"=0.0, "Speed"=0.0} ("Test"), "Target Load"=w403) -> (w405:T12)
                      n80 = Bundle By Name(cluster=w399, "Start.TUU.CP PID"=TRUE) -> (w400:T1)
                      n81 = call "Main - Set and Run PID (SubVI).vi"("Action"=T13."Run Target", "error in (no error)"=w401, "Test"=w405, "IP Address"=w404) -> ("error out"=w402:errorcluster)  [unwired: 7 in]
                    }
                    frame True {
                    }
                  }
                  n82 = And(x=w368, y=w367) -> (x .and. y?=w366:bool)
                  n83 = case shown="True" w367 {
                    tunnel: w364 -> [w381 w389]
                    tunnel: [w379 w388] -> w377
                    tunnel: w376 -> [_ w387]
                    tunnel: w374 -> [_ w386]
                    tunnel: [w378 w385] -> w371
                    tunnel: w370 -> [w378 w384]
                    tunnel: w366 -> [_ w383]
                    tunnel: w362 -> [_ w382]
                    frame False {
                      n84 = Bundle By Name(cluster=w381, "Start.TUU.PreStart"=TRUE ("Start.TS.PreStart")) -> (w379:T1)
                    }
                    frame True {
                      n85 = case shown="True" w383 {
                        tunnel: w389 -> [w393 w397]
                        tunnel: [w393 w395] -> w388
                        tunnel: w387 -> [_ _]
                        tunnel: w386 -> [_ _]
                        tunnel: [w392 w394] -> w385
                        tunnel: w384 -> [w392 w394]
                        tunnel: w382 -> [w391 _]
                        frame False {
                          n86 = call "Main - Seconds to Time (SubVI).vi"("Seconds"=w391) -> ("Time string"=w390:string)  [unwired: 9 in, 1 out]
                          n87 = local write "Delay"(w390) -> ()
                        }
                        frame True {
                          n88 = Bundle By Name(cluster=w397, "Start.TUU.PreStart"=TRUE ("Start.TS.PreStart")) -> (w395:T1)
                        }
                      }
                    }
                  }
                }
                frame True {
                  n89 = Bundle By Name(cluster=w413, "Test RunTime"=w412, "Stop.TUU.Prev Time"=w412, "Calc.TUU.MaxDeviator"=sgl 0.0, "1st Log"=TRUE, "Log Prev Time"=w412) -> (w414:T1)
                }
              }
            }
          }
        }
        frame True {
          n90 = case shown="False" w419 {
            tunnel: [w432 w436] -> w423
            tunnel: w422 -> [w431 w436]
            tunnel: w421 -> [w430 _]
            tunnel: w420 -> [w426 _]
            tunnel: [w429 w437] -> w418
            tunnel: w417 -> [w428 w437]
            frame False {
              n91 = Bundle By Name(cluster=T12 {"Target Load"=0.0, "Target Disp"=0.0, "Rate"=0.0, "Speed"=0.0} ("Test"), "Speed"=w426) -> (w435:T12)
              n92 = Bundle By Name(cluster=w428, "Start.TUU.Trig SS"=TRUE ("Start.TS.Trig SS")) -> (w429:T1)
              n93 = call "Main - Set and Run PID (SubVI).vi"("Action"=T13."Run Disp", "error in (no error)"=w431, "Test"=w435, "IP Address"=w430) -> ("error out"=w432:errorcluster)  [unwired: 7 in]
            }
            frame True {
            }
          }
          n94 = case shown="False" w424 {
            tunnel: [RunTest_-_State."Check Stop" RunTest_-_State."Check Post Stop"] -> w425
            frame False {
            }
            frame True {
            }
          }
        }
      }
    }
    frame 3 {
      n95 = Unbundle By Name(w465) -> ("StartTime"=w446:dbl, "Start.SB.Delay Value"=w443:dbl, "Start.SB.Delay"=w447:bool, "Start.SB.VS"=w452:dbl, "Start.SB.Trig SS"=w453:bool, "Stop.SB.PostStop Run"=w454:bool, "Running?"=w456:bool, "Start.SB.LC"=w462:dbl, "Start.SB.Engage"=w466:bool, "Start.SB.ES"=w467:dbl, "Start.SB.PreStart"=w469:bool, "Start.SB.SS"=w455:dbl, "Start.SB.VS PID"=w444:bool, "IP Address"=w459:string[], "KeyName"=w451:string[])
      n96 = Subtract(x=w440, y=w446) -> (x-y=w442:dbl)
      n97 = Search 1D Array(1D array=w451, element="HLC Shearbox" ("String")) -> (index of element=w460:i32)  [unwired: 1 in]
      n98 = Search 1D Array(1D array=w451, element="VLC Shearbox" ("String")) -> (index of element=w449:i32)  [unwired: 1 in]
      n99 = Subtract(x=w443, y=w442) -> (x-y=w441:dbl)
      n100 = Greater Or Equal?(x=w442, y=w443) -> (x >= y?=w445:bool)
      n101 = Index Array(array=w459, index #1=w460, index #2=w449) -> (element #1=w457:string, element #2=w448:string)
      n102 = case shown="False" w456 {
        tunnel: w469 -> [w486 _]
        tunnel: w468 -> [w485 w680]
        tunnel: w467 -> [w484 _]
        tunnel: w466 -> [w483 _]
        tunnel: w465 -> [w482 w675]
        tunnel: [w481 w676] -> w464
        tunnel: [w480 w681] -> w463
        tunnel: w462 -> [w479 _]
        tunnel: [w478 w683] -> w461
        tunnel: w457 -> [w477 w679]
        tunnel: w455 -> [_ w678]
        tunnel: w454 -> [_ w682]
        tunnel: w453 -> [_ w677]
        tunnel: w452 -> [w476 _]
        tunnel: w448 -> [w475 _]
        tunnel: w447 -> [w474 _]
        tunnel: w445 -> [w473 _]
        tunnel: w444 -> [w472 _]
        tunnel: w441 -> [w471 _]
        tunnel: w440 -> [w470 _]
        frame False {
          n103 = case shown="True" w483 {
            tunnel: w486 -> [w502 w619]
            tunnel: w485 -> [w501 w618]
            tunnel: w484 -> [w500 w617]
            tunnel: [w499 w616] -> w480
            tunnel: w482 -> [w498 w615]
            tunnel: [w497 w614] -> w481
            tunnel: w479 -> [w496 w613]
            tunnel: [w495 w612] -> w478
            tunnel: w477 -> [w494 w611]
            tunnel: w476 -> [w493 w610]
            tunnel: w475 -> [w492 w609]
            tunnel: w474 -> [w491 w608]
            tunnel: w473 -> [w490 w607]
            tunnel: w472 -> [w489 w606]
            tunnel: w471 -> [w488 w605]
            tunnel: w470 -> [w487 w604]
            frame True {
              n104 = case shown="True" w502 {
                tunnel: w501 -> [w510 w580]
                tunnel: [w512 w581] -> w499
                tunnel: w500 -> [w515 _]
                tunnel: w498 -> [w504 w571]
                tunnel: [w518 w577] -> w497
                tunnel: w496 -> [_ w578]
                tunnel: [RunTest_-_State."Idle" w582] -> w495
                tunnel: w494 -> [w517 _]
                tunnel: w493 -> [w513 w568]
                tunnel: w492 -> [w514 _]
                tunnel: w491 -> [w508 _]
                tunnel: w490 -> [w509 _]
                tunnel: w489 -> [w506 _]
                tunnel: w488 -> [w503 _]
                tunnel: w487 -> [_ w576]
                frame False {
                  n105 = case shown="False" w506 {
                    tunnel: w514 -> [w561 _]
                    tunnel: w513 -> [w560 _]
                    tunnel: [w559 w565] -> w511
                    tunnel: w510 -> [w558 w565]
                    tunnel: [w557 w566] -> w505
                    tunnel: w504 -> [w556 w566]
                    frame False {
                      n106 = Bundle By Name(cluster=T12 {"Target Load"=0.0, "Target Disp"=0.0, "Rate"=0.0, "Speed"=0.0} ("Test"), "Target Load"=w560) -> (w562:T12)
                      n107 = Bundle By Name(cluster=w556, "Start.SB.VS PID"=TRUE ("Start.TUU.CP PID")) -> (w557:T1)
                      n108 = call "Main - Set and Run PID (SubVI).vi"("Action"=T13."Run Target", "error in (no error)"=w558, "Test"=w562, "IP Address"=w561) -> ("error out"=w559:errorcluster)  [unwired: 7 in]
                    }
                    frame True {
                    }
                  }
                  n109 = And(x=w509, y=w508) -> (x .and. y?=w507:bool)
                  n110 = case shown="True" w508 {
                    tunnel: w505 -> [w526 w537]
                    tunnel: [w524 w536] -> w518
                    tunnel: w517 -> [w523 w535]
                    tunnel: w515 -> [w522 w534]
                    tunnel: [w521 w533] -> w512
                    tunnel: w511 -> [w520 w532]
                    tunnel: w507 -> [_ w531]
                    tunnel: w503 -> [_ w530]
                    frame False {
                      n111 = Bundle By Name(cluster=T12 {"Target Load"=0.0, "Target Disp"=0.0, "Rate"=0.0, "Speed"=0.0} ("Test"), "Speed"=w522) -> (w529:T12)
                      n112 = Bundle By Name(cluster=w526, "Start.SB.PreStart"=TRUE ("Start.TS.PreStart"), "1run"=TRUE) -> (w524:T1)
                      n113 = call "Main - Set and Run PID (SubVI).vi"("Action"=T13."Run Disp", "error in (no error)"=w520, "Test"=w529, "IP Address"=w523) -> ("error out"=w521:errorcluster)  [unwired: 7 in]
                    }
                    frame True {
                      n114 = case shown="False" w531 {
                        tunnel: w537 -> [w539 w551]
                        tunnel: [w540 w549] -> w536
                        tunnel: w535 -> [_ w548]
                        tunnel: w534 -> [_ w547]
                        tunnel: [w543 w546] -> w533
                        tunnel: w532 -> [w543 w545]
                        tunnel: w530 -> [w542 _]
                        frame False {
                          n115 = call "Main - Seconds to Time (SubVI).vi"("Seconds"=w542) -> ("Time string"=w541:string)  [unwired: 9 in, 1 out]
                          n116 = Bundle By Name(cluster=w539, "1run"=TRUE) -> (w540:T1)
                          n117 = local write "Delay"(w541) -> ()
                        }
                        frame True {
                          n118 = Bundle By Name(cluster=T12 {"Target Load"=0.0, "Target Disp"=0.0, "Rate"=0.0, "Speed"=0.0} ("Test"), "Speed"=w547) -> (w554:T12)
                          n119 = Bundle By Name(cluster=w551, "Start.SB.PreStart"=TRUE ("Start.TS.PreStart"), "1run"=TRUE) -> (w549:T1)
                          n120 = call "Main - Set and Run PID (SubVI).vi"("Action"=T13."Run Disp", "error in (no error)"=w545, "Test"=w554, "IP Address"=w548) -> ("error out"=w546:errorcluster)  [unwired: 7 in]
                        }
                      }
                    }
                  }
                }
                frame True {
                  w567 = 10.0 ("x")
                  n121 = Unbundle By Name(w571) -> ("Sensor Data"=w573:sgl[])
                  n122 = Unbundle By Name(w571) -> ("Calc.SB.H LC"=w579:sgl)
                  n123 = Add(x=w567, y=w568) -> (x+y=w575:dbl)
                  n124 = Subtract(x=w568, y=w567) -> (x-y=w574:dbl)
                  n125 = Index Array(array=w573) -> (element=w572:sgl)  [unwired: 1 in]
                  n126 = In Range and Coerce(upper limit=w575, x=w572, lower limit=w574) -> (In Range?=w569:bool)  [unwired: 1 out]
                  n127 = Greater Or Equal?(x=w579, y=w578) -> (x >= y?=w570:bool)
                  n128 = case shown="False" w570 {
                    tunnel: [RunTest_-_State."Idle" RunTest_-_State."Run"] -> w582
                    tunnel: [w595 w597] -> w581
                    tunnel: w580 -> [w594 w597]
                    tunnel: w579 -> [w592 _]
                    tunnel: w578 -> [w591 _]
                    tunnel: [w588 w602] -> w577
                    tunnel: w571 -> [w587 w601]
                    tunnel: w576 -> [_ w598]
                    tunnel: w569 -> [w584 _]
                    frame False {
                      # "cpt\nbpt\nvc\nlt\ndisp\nppt"
                      n129 = Unbundle By Name(w587) -> ("Calc.SB.Shear Strain"=w585:sgl)
                      n130 = Format Into String(format string="Load Change %f < %f" ("Delay"), initial string="", error in=w594, w592, w591) -> (resulting string=w586:string, error out=w595:errorcluster)
                      n131 = Not(x=w584) -> (.not. x?=w583:bool)
                      n132 = local write "Delay"(w586) -> ()
                      n133 = Bundle By Name(cluster=w587, "Log Prev Axial"=w585, "1run"=w583) -> (w588:T1)
                    }
                    frame True {
                      n134 = Bundle By Name(cluster=w601, "Test RunTime"=w598, "Stop.SB.Prev Time"=w598, "Calc.SB.MaxShear"=sgl 0.0 ("Calc.SB.MaxDeviator"), "1st Log"=TRUE, "Log Prev Time"=w598, "1run"=TRUE) -> (w602:T1)
                    }
                  }
                }
              }
            }
            frame False {
              n135 = case shown="False" w619 {
                tunnel: w618 -> [w627 w673]
                tunnel: [w629 w673] -> w616
                tunnel: w617 -> [w632 _]
                tunnel: w615 -> [w621 w671]
                tunnel: [w635 w672] -> w614
                tunnel: w613 -> [_ _]
                tunnel: [RunTest_-_State."Idle" RunTest_-_State."Run"] -> w612
                tunnel: w611 -> [w634 _]
                tunnel: w610 -> [w630 _]
                tunnel: w609 -> [w631 _]
                tunnel: w608 -> [w625 _]
                tunnel: w607 -> [w626 _]
                tunnel: w606 -> [w623 _]
                tunnel: w605 -> [w620 _]
                tunnel: w604 -> [_ w670]
                frame False {
                  n136 = case shown="False" w623 {
                    tunnel: w631 -> [w662 _]
                    tunnel: w630 -> [w661 _]
                    tunnel: [w660 w666] -> w628
                    tunnel: w627 -> [w659 w666]
                    tunnel: [w658 w667] -> w622
                    tunnel: w621 -> [w657 w667]
                    frame False {
                      n137 = Bundle By Name(cluster=T12 {"Target Load"=0.0, "Target Disp"=0.0, "Rate"=0.0, "Speed"=0.0} ("Test"), "Target Load"=w661) -> (w663:T12)
                      n138 = Bundle By Name(cluster=w657, "Start.SB.VS PID"=TRUE ("Start.TUU.CP PID")) -> (w658:T1)
                      n139 = call "Main - Set and Run PID (SubVI).vi"("Action"=T13."Run Target", "error in (no error)"=w659, "Test"=w663, "IP Address"=w662) -> ("error out"=w660:errorcluster)  [unwired: 7 in]
                    }
                    frame True {
                    }
                  }
                  n140 = And(x=w626, y=w625) -> (x .and. y?=w624:bool)
                  n141 = case shown="True" w625 {
                    tunnel: w622 -> [w639 w647]
                    tunnel: [w637 w646] -> w635
                    tunnel: w634 -> [_ w645]
                    tunnel: w632 -> [_ w644]
                    tunnel: [w636 w643] -> w629
                    tunnel: w628 -> [w636 w642]
                    tunnel: w624 -> [_ w641]
                    tunnel: w620 -> [_ w640]
                    frame False {
                      n142 = Bundle By Name(cluster=w639, "Start.SB.PreStart"=TRUE ("Start.TS.PreStart")) -> (w637:T1)
                    }
                    frame True {
                      n143 = case shown="True" w641 {
                        tunnel: w647 -> [w651 w655]
                        tunnel: [w651 w653] -> w646
                        tunnel: w645 -> [_ _]
                        tunnel: w644 -> [_ _]
                        tunnel: [w650 w652] -> w643
                        tunnel: w642 -> [w650 w652]
                        tunnel: w640 -> [w649 _]
                        frame False {
                          n144 = call "Main - Seconds to Time (SubVI).vi"("Seconds"=w649) -> ("Time string"=w648:string)  [unwired: 9 in, 1 out]
                          n145 = local write "Delay"(w648) -> ()
                        }
                        frame True {
                          n146 = Bundle By Name(cluster=w655, "Start.SB.PreStart"=TRUE ("Start.TS.PreStart")) -> (w653:T1)
                        }
                      }
                    }
                  }
                }
                frame True {
                  n147 = Bundle By Name(cluster=w671, "Test RunTime"=w670, "Stop.SB.Prev Time"=w670, "Calc.SB.MaxShear"=sgl 0.0 ("Calc.SB.MaxDeviator"), "1st Log"=TRUE, "Log Prev Time"=w670) -> (w672:T1)
                }
              }
            }
          }
        }
        frame True {
          n148 = case shown="False" w677 {
            tunnel: [w690 w694] -> w681
            tunnel: w680 -> [w689 w694]
            tunnel: w679 -> [w688 _]
            tunnel: w678 -> [w684 _]
            tunnel: [w687 w695] -> w676
            tunnel: w675 -> [w686 w695]
            frame False {
              n149 = Bundle By Name(cluster=T12 {"Target Load"=0.0, "Target Disp"=0.0, "Rate"=0.0, "Speed"=0.0} ("Test"), "Speed"=w684) -> (w693:T12)
              n150 = Bundle By Name(cluster=w686, "Start.SB.Trig SS"=TRUE ("Start.TS.Trig SS")) -> (w687:T1)
              n151 = call "Main - Set and Run PID (SubVI).vi"("Action"=T13."Run Disp", "error in (no error)"=w689, "Test"=w693, "IP Address"=w688) -> ("error out"=w690:errorcluster)  [unwired: 7 in]
            }
            frame True {
            }
          }
          n152 = case shown="False" w682 {
            tunnel: [RunTest_-_State."Check Stop" RunTest_-_State."Check Post Stop"] -> w683
            frame False {
            }
            frame True {
            }
          }
        }
      }
    }
    frame 4 {
      n153 = Unbundle By Name(w707) -> ("Stop.Perm.PostStop Run"=w698:bool, "Stop.Perm.RatioTime"=w699:dbl, "Stop.Perm.Ratio"=w700:bool, "Stop.Perm.Time"=w706:dbl, "Stop.Perm.Max Time"=w701:bool, "Running?"=w711:bool, "IP Address"=w710:string[], "Start.Perm.DP"=w709:dbl, "KeyName"=w705:string[])
      n154 = Search 1D Array(1D array=w705, element="BPC2 Permeability" ("String")) -> (index of element=w703:i32)  [unwired: 1 in]
      n155 = case shown="False" w711 {
        tunnel: [w725 w761] -> w714
        tunnel: w713 -> [w727 w761]
        tunnel: w710 -> [w731 _]
        tunnel: w709 -> [w723 _]
        tunnel: [RunTest_-_State."Run" w760] -> w712
        tunnel: [w729 w762] -> w708
        tunnel: w707 -> [w724 w762]
        tunnel: w706 -> [w730 _]
        tunnel: w703 -> [w728 _]
        tunnel: w702 -> [w721 _]
        tunnel: w701 -> [w718 _]
        tunnel: w700 -> [w719 _]
        tunnel: w699 -> [w715 _]
        tunnel: w698 -> [_ w759]
        frame False {
          n156 = Index Array(array=w731, index=w728) -> (element=w726:string)
          n157 = for {
            N: 3 -> [_]
            tunnel: w726 -> [w736]
            tunnel: w723 -> [w732]
            shift-right: [w733] -> w725
            shift-left: w727 -> [w738]
            n158 = Bundle By Name(cluster=T12 {"Target Load"=0.0, "Target Disp"=0.0, "Rate"=0.0, "Speed"=0.0} ("Test"), "Target Load"=w732) -> (w734:T12)
            n159 = call "Main - Set and Run PID (SubVI).vi"("Action"=T13."Run Target", "error in (no error)"=w738, "Test"=w734, "IP Address"=w736) -> ("error out"=w733:errorcluster)  [unwired: 7 in]
          }
          n160 = Build Array(w719, w718) -> (w717:bool[])
          n161 = Boolean Array To Number(Boolean array=w717) -> (number=w716:u32)
          n162 = case shown="3" w716 {
            tunnel: w721 -> [w739 w743 w748 w754]
            tunnel: w730 -> [_ _ w751 w758]
            tunnel: [w741 w746 w750 w757] -> w729
            tunnel: w724 -> [w740 w745 w747 w755]
            tunnel: w715 -> [_ w742 _ w753]
            frame 0, Default {
              n163 = Bundle By Name(cluster=w740, "Test RunTime"=w739, "Log Prev Time"=w739) -> (w741:T1)
            }
            frame 1 {
              n164 = Add(x=w742, y=w743) -> (x+y=w744:dbl)
              n165 = Bundle By Name(cluster=w745, "Stop.Perm.Time Cond 2"=w744, "Test RunTime"=w743, "Log Prev Time"=w743) -> (w746:T1)
            }
            frame 2 {
              n166 = Add(x=w751, y=w748) -> (x+y=w749:dbl)
              n167 = Bundle By Name(cluster=w747, "Stop.Perm.Time Cond"=w749, "Test RunTime"=w748, "Log Prev Time"=w748) -> (w750:T1)
            }
            frame 3 {
              n168 = Add(x=w753, y=w754) -> (x+y=w752:dbl)
              n169 = Add(x=w758, y=w754) -> (x+y=w756:dbl)
              n170 = Bundle By Name(cluster=w755, "Stop.Perm.Time Cond 2"=w752, "Stop.Perm.Time Cond"=w756, "Test RunTime"=w754, "Log Prev Time"=w754) -> (w757:T1)
            }
          }
        }
        frame True {
          n171 = case shown="False" w759 {
            tunnel: [RunTest_-_State."Check Stop" RunTest_-_State."Check Post Stop"] -> w760
            frame False {
            }
            frame True {
            }
          }
        }
      }
    }
    frame 5 {
      n172 = Unbundle By Name(w772) -> ("Stop.Cons.Select"=w770:i32, "Stop.Cons.Time"=w771:dbl, "Start.Cons.Delay"=w781:bool, "Start.Cons.No Delay"=w780:dbl, "Running?"=w776:bool, "IP Address"=w775:string[], "Start.Cons.VS"=w774:dbl, "StartTime"=w769:dbl, "KeyName"=w768:string[])
      n173 = Search 1D Array(1D array=w768, element="VLC Consolidation" ("String")) -> (index of element=w766:i32)  [unwired: 1 in]
      n174 = case shown="False" w781 {
        tunnel: w780 -> [w783 _]
        tunnel: [w797 w888] -> w779
        tunnel: w778 -> [w787 w889]
        tunnel: [w796 w884] -> w777
        tunnel: w776 -> [w795 w887]
        tunnel: w775 -> [w794 w886]
        tunnel: w774 -> [w793 w885]
        tunnel: [w792 w883] -> w773
        tunnel: w772 -> [w791 w882]
        tunnel: w771 -> [w790 w881]
        tunnel: w770 -> [w789 w879]
        tunnel: w769 -> [w788 _]
        tunnel: w766 -> [w785 w880]
        tunnel: w765 -> [w782 w878]
        frame True {
          n175 = Subtract(x=w782, y=w788) -> (x-y=w784:dbl)
          n176 = Greater?(x=w784, y=w783) -> (0:w786:bool)
          n177 = case shown="False" w786 {
            tunnel: [w804 w816] -> w797
            tunnel: w787 -> [w804 w815]
            tunnel: [RunTest_-_State."Idle" w812] -> w796
            tunnel: w795 -> [_ w817]
            tunnel: w794 -> [_ w814]
            tunnel: w793 -> [_ w813]
            tunnel: [w802 w811] -> w792
            tunnel: w791 -> [w802 w810]
            tunnel: w790 -> [_ w809]
            tunnel: w789 -> [_ w808]
            tunnel: w785 -> [_ w807]
            tunnel: w783 -> [w799 w806]
            tunnel: w784 -> [w801 _]
            tunnel: w782 -> [_ w805]
            frame False {
              n178 = Subtract(x=w799, y=w801) -> (x-y=w800:dbl)
              n179 = call "Main - Seconds to Time (SubVI).vi"("Seconds"=w800) -> ("Time string"=w798:string)  [unwired: 9 in, 1 out]
              n180 = local write "Delay"(w798) -> ()
            }
            frame True {
              n181 = case shown="False" w817 {
                tunnel: [w823 w853] -> w816
                tunnel: w815 -> [w825 w852]
                tunnel: w814 -> [w830 w850]
                tunnel: w813 -> [w821 w851]
                tunnel: [RunTest_-_State."Run" RunTest_-_State."Check Stop"] -> w812
                tunnel: [w828 w854] -> w811
                tunnel: w810 -> [w822 w854]
                tunnel: w809 -> [w829 _]
                tunnel: w808 -> [w827 _]
                tunnel: w807 -> [w826 w849]
                tunnel: w806 -> [_ _]
                tunnel: w805 -> [w819 _]
                frame False {
                  n182 = Index Array(array=w830, index=w826) -> (element=w824:string)
                  n183 = for {
                    N: 3 -> [_]
                    tunnel: w824 -> [w833]
                    tunnel: w821 -> [w831]
                    shift-right: [w832] -> w823
                    shift-left: w825 -> [w834]
                    n184 = Bundle By Name(cluster=T12 {"Target Load"=0.0, "Target Disp"=0.0, "Rate"=0.0, "Speed"=0.0} ("Test"), "Target Load"=w831) -> (w837:T12)
                    n185 = call "Main - Set and Run PID (SubVI).vi"("Action"=T13."Run Target", "error in (no error)"=w834, "Test"=w837, "IP Address"=w833) -> ("error out"=w832:errorcluster)  [unwired: 7 in]
                  }
                  n186 = case shown="1" w827 {
                    tunnel: w819 -> [w842 w846]
                    tunnel: w829 -> [w844 _]
                    tunnel: [w843 w848] -> w828
                    tunnel: w822 -> [w841 w847]
                    frame 0, Default {
                      n187 = Unbundle By Name(w841) -> ("Sensor Data"=w840:sgl[])
                      n188 = Index Array(array=w840, index=1) -> (element=w838:sgl)
                      n189 = Add(x=w844, y=w842) -> (x+y=w845:dbl)
                      n190 = Bundle By Name(cluster=w841, "Stop.Cons.Last Disp"=w838, "Stop.Cons.Time Cond"=w845, "Test RunTime"=w842, "Log Prev Time"=w842) -> (w843:T1)
                    }
                    frame 1 {
                      n191 = Bundle By Name(cluster=w847, "Stop.Cons.Time Cond"=w846, "Test RunTime"=w846, "Log Prev Time"=w846) -> (w848:T1)
                    }
                  }
                }
                frame True {
                  n192 = disable-structure shown="Disabled" {
                    disable-tunnel: w854 -> [w863 _]
                    disable-tunnel: [w862 w877] -> w853
                    disable-tunnel: w852 -> [w861 w877]
                    disable-tunnel: w851 -> [w860 _]
                    disable-tunnel: w850 -> [w859 _]
                    disable-tunnel: w849 -> [w858 _]
                    frame Disabled {
                      n193 = Unbundle By Name(w863) -> ("Sensor Data"=w866:sgl[])
                      n194 = Index Array(array=w866) -> (element=w856:sgl)  [unwired: 1 in]
                      n195 = Increment(x=w860) -> (x+1=w864:dbl)
                      n196 = Decrement(x=w860) -> (x-1=w865:dbl)
                      n197 = In Range and Coerce(upper limit=w864, x=w856, lower limit=w865) -> (In Range?=w857:bool)  [unwired: 1 out]
                      n198 = case shown="False" w857 {
                        tunnel: [w871 w876] -> w862
                        tunnel: w861 -> [w870 w876]
                        tunnel: w860 -> [w869 _]
                        tunnel: w859 -> [w868 _]
                        tunnel: w858 -> [w867 _]
                        frame False {
                          n199 = Bundle By Name(cluster=T12 {"Target Load"=0.0, "Target Disp"=0.0, "Rate"=0.0, "Speed"=0.0} ("Test"), "Target Load"=w869) -> (w875:T12)
                          n200 = Index Array(array=w868, index=w867) -> (element=w872:string)
                          n201 = call "Main - Set and Run PID (SubVI).vi"("Action"=T13."Run Target", "error in (no error)"=w870, "Test"=w875, "IP Address"=w872) -> ("error out"=w871:errorcluster)  [unwired: 7 in]
                        }
                        frame True {
                        }
                      }
                    }
                    frame Enabled {
                    }
                  }
                }
              }
            }
          }
        }
        frame False {
          n202 = case shown="False" w887 {
            tunnel: [w895 w925] -> w888
            tunnel: w889 -> [w898 w924]
            tunnel: w886 -> [w902 w922]
            tunnel: w885 -> [w893 w923]
            tunnel: [RunTest_-_State."Run" RunTest_-_State."Check Stop"] -> w884
            tunnel: [w900 w926] -> w883
            tunnel: w882 -> [w894 w926]
            tunnel: w881 -> [w901 _]
            tunnel: w880 -> [w899 w921]
            tunnel: w879 -> [w896 _]
            tunnel: w878 -> [w891 _]
            frame False {
              n203 = Index Array(array=w902, index=w899) -> (element=w897:string)
              n204 = for {
                N: 3 -> [_]
                tunnel: w897 -> [w907]
                tunnel: w893 -> [w903]
                shift-right: [w904] -> w895
                shift-left: w898 -> [w909]
                n205 = Bundle By Name(cluster=T12 {"Target Load"=0.0, "Target Disp"=0.0, "Rate"=0.0, "Speed"=0.0} ("Test"), "Target Load"=w903) -> (w905:T12)
                n206 = call "Main - Set and Run PID (SubVI).vi"("Action"=T13."Run Target", "error in (no error)"=w909, "Test"=w905, "IP Address"=w907) -> ("error out"=w904:errorcluster)  [unwired: 7 in]
              }
              n207 = case shown="0, Default" w896 {
                tunnel: w891 -> [w914 w918]
                tunnel: w901 -> [w917 _]
                tunnel: [w916 w920] -> w900
                tunnel: w894 -> [w913 w919]
                frame 0, Default {
                  n208 = Unbundle By Name(w913) -> ("Sensor Data"=w912:sgl[])
                  n209 = Index Array(array=w912, index=1) -> (element=w911:sgl)
                  n210 = Add(x=w917, y=w914) -> (x+y=w915:dbl)
                  n211 = Bundle By Name(cluster=w913, "Stop.Cons.Last Disp"=w911, "Stop.Cons.Time Cond"=w915, "Test RunTime"=w914, "Log Prev Time"=w914) -> (w916:T1)
                }
                frame 1 {
                  n212 = Bundle By Name(cluster=w919, "Stop.Cons.Time Cond"=w918, "Test RunTime"=w918, "Log Prev Time"=w918) -> (w920:T1)
                }
              }
            }
            frame True {
              n213 = disable-structure shown="Disabled" {
                disable-tunnel: w926 -> [w938 _]
                disable-tunnel: [w937 w949] -> w925
                disable-tunnel: w924 -> [w936 w949]
                disable-tunnel: w923 -> [w935 _]
                disable-tunnel: w922 -> [w934 _]
                disable-tunnel: w921 -> [w933 _]
                frame Disabled {
                  n214 = Unbundle By Name(w938) -> ("Sensor Data"=w932:sgl[])
                  n215 = Index Array(array=w932) -> (element=w928:sgl)  [unwired: 1 in]
                  n216 = Increment(x=w935) -> (x+1=w930:dbl)
                  n217 = Decrement(x=w935) -> (x-1=w931:dbl)
                  n218 = In Range and Coerce(upper limit=w930, x=w928, lower limit=w931) -> (In Range?=w929:bool)  [unwired: 1 out]
                  n219 = case shown="False" w929 {
                    tunnel: [w943 w948] -> w937
                    tunnel: w936 -> [w942 w948]
                    tunnel: w935 -> [w941 _]
                    tunnel: w934 -> [w940 _]
                    tunnel: w933 -> [w939 _]
                    frame False {
                      n220 = Index Array(array=w940, index=w939) -> (element=w946:string)
                      n221 = Bundle By Name(cluster=T12 {"Target Load"=0.0, "Target Disp"=0.0, "Rate"=0.0, "Speed"=0.0} ("Test"), "Target Load"=w941) -> (w944:T12)
                      n222 = call "Main - Set and Run PID (SubVI).vi"("Action"=T13."Run Target", "error in (no error)"=w942, "Test"=w944, "IP Address"=w946) -> ("error out"=w943:errorcluster)  [unwired: 7 in]
                    }
                    frame True {
                    }
                  }
                }
                frame Enabled {
                }
              }
            }
          }
        }
      }
    }
    frame 6 {
      n223 = Unbundle By Name(w951) -> ("PreStart Sat"=w950:bool)
      n224 = case shown="False" w950 {
        tunnel: [w970 w1055] -> w956
        tunnel: w955 -> [w971 w1054]
        tunnel: [RunTest_-_State."Idle" w1053] -> w954
        tunnel: [w969 w1050] -> w953
        tunnel: w951 -> [w968 w1049]
        tunnel: w952 -> [_ w1042]
        frame False {
          n225 = Unbundle By Name(w968) -> ("Sensor Data"=w973:sgl[], "Start.Sat.CP"=w960:dbl, "Start.Sat.BP"=w959:dbl)
          n226 = Index Array(array=w973) -> (element #1=w961:sgl, element #2=w957:sgl, element #4=w958:sgl)  [unwired: 4 in, 1 out]
          n227 = Less?(x=w961, y=w960) -> (x < y?=w964:bool)
          n228 = Less?(x=w957, y=w959) -> (x < y?=w965:bool)
          n229 = Less?(x=w958, y=w959) -> (x < y?=w966:bool)
          n230 = Subtract(x=w957, y=w961) -> (x-y=w962:sgl)
          n231 = Less Or Equal?(x=w962, y=sgl 5.0) -> (x <= y?=w963:bool)
          n232 = Compound Arithmetic op=AND(w963, w964, w965, w966) -> (w972:bool)
          n233 = case shown="False" w972 {
            selector: w972 -> [_ w1036]
            tunnel: [w999 w1038] -> w969
            tunnel: w968 -> [w999 w1037]
            tunnel: [w989 w1035] -> w970
            tunnel: w971 -> [w997 w1035]
            tunnel: w966 -> [w994 _]
            tunnel: w965 -> [w993 _]
            tunnel: w964 -> [w992 _]
            tunnel: w963 -> [w991 _]
            tunnel: w962 -> [w980 _]
            tunnel: w961 -> [w979 _]
            tunnel: w960 -> [w978 _]
            tunnel: w957 -> [w977 _]
            tunnel: w959 -> [w975 _]
            tunnel: w958 -> [w976 _]
            frame False {
              n234 = case shown="False" w994 {
                tunnel: [w1004 w1007] -> w996
                tunnel: w997 -> [w1005 w1007]
                tunnel: [w1003 ""] -> w985
                tunnel: w976 -> [w1001 _]
                tunnel: w975 -> [w1000 _]
                frame False {
                  n235 = Format Into String(format string="PWP < Target BP = %f<%f ; " ("message"), initial string="", error in=w1005, w1001, w1000) -> (resulting string=w1003:string, error out=w1004:errorcluster)
                }
                frame True {
                }
              }
              n236 = case shown="False" w993 {
                tunnel: [w1013 w1016] -> w995
                tunnel: w996 -> [w1014 w1016]
                tunnel: [w1011 ""] -> w986
                tunnel: w977 -> [w1010 _]
                tunnel: w975 -> [w1009 _]
                frame False {
                  n237 = Format Into String(format string="BP < Target BP = %f<%f ; " ("message"), initial string="", error in=w1014, w1010, w1009) -> (resulting string=w1011:string, error out=w1013:errorcluster)
                }
                frame True {
                }
              }
              n238 = case shown="False" w992 {
                tunnel: [w1021 w1025] -> w998
                tunnel: w995 -> [w1022 w1025]
                tunnel: [w1020 ""] -> w987
                tunnel: w979 -> [w1019 _]
                tunnel: w978 -> [w1018 _]
                frame False {
                  n239 = Format Into String(format string="CP < Target CP = %f<%f ; " ("message"), initial string="", error in=w1022, w1019, w1018) -> (resulting string=w1020:string, error out=w1021:errorcluster)
                }
                frame True {
                }
              }
              n240 = case shown="False" w991 {
                tunnel: [w1030 w1033] -> w990
                tunnel: w998 -> [w1031 w1033]
                tunnel: [w1028 ""] -> w988
                tunnel: w980 -> [w1027 _]
                frame False {
                  n241 = Format Into String(format string="BP - CP < 5 = %f ; " ("message"), initial string="", error in=w1031, w1027) -> (resulting string=w1028:string, error out=w1030:errorcluster)
                }
                frame True {
                }
              }
              n242 = Concatenate Strings(w988, w987, w986, w985) -> (w984:string)
              n243 = Format Into String(format string="Action Required\nOne or more of the instrument parameters are beyond normal range required to initiate the test. (%s)" ("message"), initial string="", error in=w990, w984) -> (resulting string=w982:string, error out=w989:errorcluster)
              n244 = One Button Dialog(message=w982) -> ()  [unwired: 1 in, 1 out]
            }
            frame True {
              n245 = Bundle By Name(cluster=w1037, "PreStart Sat"=w1036) -> (w1038:T1)
            }
          }
        }
        frame True {
          # "cpt\nbpt\nvc\nppt"
          n246 = Unbundle By Name(w1049) -> ("Start.Sat.Target BP"=w1039:bool, "Start.Sat.Target CP"=w1040:bool, "Start.Sat.StartBP"=w1041:bool, "Stop.Sat.Select"=w1045:i32, "Start.Sat.CP"=w1044:dbl, "Start.Sat.BP"=w1043:dbl, "Running?"=w1052:bool, "IP Address"=w1051:string[], "KeyName"=w1048:string[])
          n247 = Build Array(w1044, w1043) -> (w1046:dbl[])
          n248 = case shown="False" w1052 {
            tunnel: [w1063 w1141] -> w1055
            tunnel: w1054 -> [w1070 w1140]
            tunnel: w1051 -> [w1069 w1138]
            tunnel: [RunTest_-_State."Run" w1131] -> w1053
            tunnel: [w1068 w1134] -> w1050
            tunnel: w1049 -> [w1062 w1142]
            tunnel: w1048 -> [w1066 w1139]
            tunnel: string[] ["CPC Saturation", "BPC Saturation"] -> [w1067 w1137]
            tunnel: w1046 -> [w1065 w1136]
            tunnel: w1045 -> [w1064 _]
            tunnel: w1042 -> [w1057 _]
            tunnel: w1041 -> [w1056 w1135]
            tunnel: w1040 -> [_ w1133]
            tunnel: w1039 -> [_ w1132]
            frame False {
              n249 = Unbundle By Name(w1062) -> ("Sensor Data"=w1061:sgl[])
              n250 = case shown="True" w1056 {
                tunnel: w1070 -> [w1083 w1096]
                tunnel: w1069 -> [w1082 w1095]
                tunnel: w1067 -> [w1076 w1094]
                tunnel: w1066 -> [w1081 w1093]
                tunnel: w1065 -> [w1072 w1092]
                tunnel: [w1080 w1091] -> w1063
                frame True {
                  n251 = Index Array(array=w1076, index=0) -> (element=w1075:string)
                  n252 = Search 1D Array(1D array=w1081, element=w1075) -> (index of element=w1078:i32)  [unwired: 1 in]
                  n253 = Index Array(array=w1082, index=w1078) -> (element=w1079:string)
                  n254 = Index Array(array=w1072, index=0) -> (element=w1071:dbl)
                  n255 = for {
                    N: 3 -> [_]
                    tunnel: w1079 -> [w1089]
                    tunnel: w1071 -> [w1084]
                    shift-right: [w1088] -> w1080
                    shift-left: w1083 -> [w1090]
                    n256 = Bundle By Name(cluster=T12 {"Target Load"=0.0, "Target Disp"=0.0, "Rate"=0.0, "Speed"=0.0} ("Test"), "Target Load"=w1084) -> (w1085:T12)
                    n257 = call "Main - Set and Run PID (SubVI).vi"("Action"=T13."Run Target", "error in (no error)"=w1090, "Test"=w1085, "IP Address"=w1089) -> ("error out"=w1088:errorcluster)  [unwired: 7 in]
                  }
                }
                frame False {
                  n258 = for {
                    tunnel: w1095 -> [w1105]
                    shift-right: [w1103] -> w1091
                    shift-left: w1096 -> [w1106]
                    tunnel: w1094 -> [w1101] mode=indexing
                    tunnel: w1093 -> [w1102]
                    tunnel: w1092 -> [w1099] mode=indexing
                    n259 = Search 1D Array(1D array=w1102, element=w1101) -> (index of element=w1100:i32)  [unwired: 1 in]
                    n260 = Index Array(array=w1105, index=w1100) -> (element=w1104:string)
                    n261 = Wait (ms)(milliseconds to wait=u32 1000) -> ()  [unwired: 1 out]
                    n262 = for {
                      N: 3 -> [_]
                      tunnel: w1104 -> [w1112]
                      tunnel: w1099 -> [w1107]
                      shift-right: [w1111] -> w1103
                      shift-left: w1106 -> [w1113]
                      n263 = Bundle By Name(cluster=T12 {"Target Load"=0.0, "Target Disp"=0.0, "Rate"=0.0, "Speed"=0.0} ("Test"), "Target Load"=w1107) -> (w1108:T12)
                      n264 = call "Main - Set and Run PID (SubVI).vi"("Action"=T13."Run Target", "error in (no error)"=w1113, "Test"=w1108, "IP Address"=w1112) -> ("error out"=w1111:errorcluster)  [unwired: 7 in]
                    }
                  }
                }
              }
              n265 = Index Array(array=w1061) -> (element #3=w1060:sgl, element #4=w1059:sgl)  [unwired: 4 in, 2 out]
              n266 = case shown="0, Default" w1064 {
                tunnel: w1057 -> [w1115 w1121 w1126]
                tunnel: [w1119 w1125 w1130] -> w1068
                tunnel: w1062 -> [w1117 w1123 w1128]
                tunnel: w1060 -> [_ w1120 _]
                tunnel: w1059 -> [w1114 _ _]
                frame 0, Default {
                  n267 = Unbundle By Name(w1117) -> ("Stop.Sat.Time"=w1116:dbl)
                  n268 = Add(x=w1116, y=w1115) -> (x+y=w1118:dbl)
                  n269 = Bundle By Name(cluster=w1117, "Stop.Sat.Last PP"=w1114, "Stop.Sat.Time Cond"=w1118, "Test RunTime"=w1115, "Log Prev Time"=w1115) -> (w1119:T1)
                }
                frame 1 {
                  n270 = Unbundle By Name(w1123) -> ("Stop.Sat.Time2"=w1122:dbl)
                  n271 = Add(x=w1122, y=w1121) -> (x+y=w1124:dbl)
                  n272 = Bundle By Name(cluster=w1123, "Stop.Sat.Last Vc"=w1120, "Stop.Sat.Time Cond 2"=w1124, "Test RunTime"=w1121, "Log Prev Time"=w1121) -> (w1125:T1)
                }
                frame 2 {
                  n273 = Unbundle By Name(w1128) -> ("Stop.Sat.Time3"=w1127:dbl)
                  n274 = Add(x=w1127, y=w1126) -> (x+y=w1129:dbl)
                  n275 = Bundle By Name(cluster=w1128, "Stop.Sat.Time Cond 3"=w1129, "Test RunTime"=w1126, "Log Prev Time"=w1126) -> (w1130:T1)
                }
              }
            }
            frame True {
              n276 = case shown="False" w1135 {
                tunnel: w1142 -> [w1144 w1150]
                tunnel: [w1145 w1156] -> w1141
                tunnel: w1140 -> [w1145 w1155]
                tunnel: w1139 -> [_ w1154]
                tunnel: w1138 -> [_ w1153]
                tunnel: w1137 -> [_ w1152]
                tunnel: w1136 -> [_ w1151]
                tunnel: [w1144 w1149] -> w1134
                tunnel: w1133 -> [_ w1148]
                tunnel: w1132 -> [_ w1147]
                tunnel: [RunTest_-_State."Check Stop" w1146] -> w1131
                frame False {
                }
                frame True {
                  n277 = case shown="False" w1148 {
                    tunnel: [w1174 w1200] -> w1156
                    tunnel: w1155 -> [w1173 w1201]
                    tunnel: w1154 -> [w1172 _]
                    tunnel: w1153 -> [w1171 _]
                    tunnel: w1152 -> [w1170 _]
                    tunnel: w1151 -> [w1168 w1204]
                    tunnel: w1150 -> [w1160 w1203]
                    tunnel: [w1159 w1202] -> w1149
                    tunnel: w1147 -> [_ w1199]
                    tunnel: [RunTest_-_State."Idle" w1198] -> w1146
                    frame False {
                      n278 = Unbundle By Name(w1160) -> ("Sensor Data"=w1169:sgl[])
                      n279 = Index Array(array=w1169, index=0) -> (element=w1166:sgl)
                      n280 = Index Array(array=w1168, index #1=0 ("index")) -> (element #1=w1165:dbl, element #2=w1161:dbl)  [unwired: 1 in]
                      n281 = Increment(x=w1165) -> (x+1=w1164:dbl)
                      n282 = Decrement(x=w1165) -> (x-1=w1163:dbl)
                      n283 = In Range and Coerce(upper limit=w1164, x=w1166, lower limit=w1163) -> (In Range?=w1162:bool)  [unwired: 1 out]
                      n284 = case shown="True" w1162 {
                        tunnel: [w1176 w1190] -> w1174
                        tunnel: w1173 -> [w1176 w1189]
                        tunnel: w1172 -> [_ w1188]
                        tunnel: w1171 -> [_ w1187]
                        tunnel: w1170 -> [_ w1183]
                        tunnel: w1161 -> [_ w1186]
                        tunnel: w1160 -> [w1175 w1180]
                        tunnel: [w1175 w1179] -> w1159
                        frame False {
                        }
                        frame True {
                          n285 = Index Array(array=w1183, index=1) -> (element=w1182:string)
                          n286 = Bundle By Name(cluster=w1180, "Start.Sat.Target CP"=TRUE ("Start.Sat.Target")) -> (w1179:T1)
                          n287 = Search 1D Array(1D array=w1188, element=w1182) -> (index of element=w1184:i32)  [unwired: 1 in]
                          n288 = Index Array(array=w1187, index=w1184) -> (element=w1185:string)
                          n289 = for {
                            N: 3 -> [_]
                            tunnel: w1186 -> [w1195]
                            tunnel: w1185 -> [w1194]
                            shift-right: [w1197] -> w1190
                            shift-left: w1189 -> [w1196]
                            n290 = Bundle By Name(cluster=T12 {"Target Load"=0.0, "Target Disp"=0.0, "Rate"=0.0, "Speed"=0.0} ("Test"), "Target Load"=w1195) -> (w1191:T12)
                            n291 = call "Main - Set and Run PID (SubVI).vi"("Action"=T13."Run Target", "error in (no error)"=w1196, "Test"=w1191, "IP Address"=w1194) -> ("error out"=w1197:errorcluster)  [unwired: 7 in]
                          }
                        }
                      }
                    }
                    frame True {
                      n292 = case shown="False" w1199 {
                        tunnel: w1204 -> [w1212 _]
                        tunnel: w1203 -> [w1210 w1229]
                        tunnel: [w1209 w1229] -> w1202
                        tunnel: w1201 -> [w1208 w1228]
                        tunnel: [w1207 w1228] -> w1200
                        tunnel: [w1205 RunTest_-_State."Check Stop"] -> w1198
                        frame False {
                          n293 = Unbundle By Name(w1210) -> ("Sensor Data"=w1218:sgl[])
                          n294 = Index Array(array=w1218, index=1) -> (element=w1216:sgl)
                          n295 = Index Array(array=w1212, index=1) -> (element=w1215:dbl)
                          n296 = Increment(x=w1215) -> (x+1=w1214:dbl)
                          n297 = Decrement(x=w1215) -> (x-1=w1213:dbl)
                          n298 = In Range and Coerce(upper limit=w1214, x=w1216, lower limit=w1213) -> (In Range?=w1206:bool)  [unwired: 1 out]
                          n299 = case shown="True" w1206 {
                            tunnel: [w1221 w1223] -> w1207
                            tunnel: w1208 -> [w1221 w1223]
                            tunnel: w1210 -> [w1220 w1226]
                            tunnel: [w1220 w1225] -> w1209
                            tunnel: [RunTest_-_State."Idle" RunTest_-_State."Check Stop"] -> w1205
                            frame False {
                            }
                            frame True {
                              n300 = Bundle By Name(cluster=w1226, "Start.Sat.Target BP"=TRUE ("Start.Sat.Target")) -> (w1225:T1)
                            }
                          }
                        }
                        frame True {
                        }
                      }
                    }
                  }
                }
              }
            }
          }
        }
      }
    }
    frame 8 {
      n301 = Unbundle By Name(w1244) -> ("Start.UCT.Trig SS"=w1231:bool, "Stop.UCT.PostStop Run"=w1232:bool, "Running?"=w1234:bool, "Start.UCT.LC"=w1241:dbl, "Start.UCT.Engage"=w1245:bool, "Start.UCT.ES"=w1246:dbl, "Start.UCT.PreStart"=w1248:bool, "Start.UCT.SS"=w1233:dbl, "IP Address"=w1238:string[], "KeyName"=w1237:string[])
      n302 = Search 1D Array(1D array=w1237, element="VLC UCT" ("String")) -> (index of element=w1239:i32)  [unwired: 1 in]
      n303 = Index Array(array=w1238, index=w1239) -> (element=w1235:string)
      n304 = case shown="False" w1234 {
        tunnel: w1248 -> [w1259 _]
        tunnel: w1247 -> [w1258 w1336]
        tunnel: w1246 -> [w1257 _]
        tunnel: w1245 -> [w1256 _]
        tunnel: w1244 -> [w1255 w1331]
        tunnel: [w1254 w1332] -> w1243
        tunnel: [w1253 w1337] -> w1242
        tunnel: w1241 -> [w1252 _]
        tunnel: [w1251 w1339] -> w1240
        tunnel: w1235 -> [w1250 w1335]
        tunnel: w1233 -> [_ w1334]
        tunnel: w1232 -> [_ w1338]
        tunnel: w1231 -> [_ w1333]
        tunnel: w1230 -> [w1249 _]
        frame False {
          n305 = case shown="True" w1256 {
            tunnel: w1259 -> [w1269 w1318]
            tunnel: w1258 -> [w1268 w1317]
            tunnel: w1257 -> [w1267 w1316]
            tunnel: [w1266 w1315] -> w1253
            tunnel: w1255 -> [w1265 w1314]
            tunnel: [w1264 w1313] -> w1254
            tunnel: w1252 -> [w1263 w1312]
            tunnel: [w1262 w1311] -> w1251
            tunnel: w1250 -> [w1261 w1310]
            tunnel: w1249 -> [w1260 w1309]
            frame True {
              n306 = case shown="True" w1269 {
                tunnel: w1268 -> [w1277 w1288]
                tunnel: [w1276 w1289] -> w1266
                tunnel: w1267 -> [w1270 _]
                tunnel: w1265 -> [w1275 w1282]
                tunnel: [w1273 w1283] -> w1264
                tunnel: w1263 -> [_ w1286]
                tunnel: [RunTest_-_State."Idle" w1290] -> w1262
                tunnel: w1261 -> [w1272 w1284]
                tunnel: w1260 -> [_ w1281]
                frame False {
                  n307 = Bundle By Name(cluster=T12 {"Target Load"=0.0, "Target Disp"=0.0, "Rate"=0.0, "Speed"=0.0} ("Test"), "Speed"=w1270) -> (w1280:T12)
                  n308 = Bundle By Name(cluster=w1275, "Start.UCT.PreStart"=TRUE ("Start.TS.PreStart")) -> (w1273:T1)
                  n309 = call "Main - Set and Run PID (SubVI).vi"("Action"=T13."Run Disp", "error in (no error)"=w1277, "Test"=w1280, "IP Address"=w1272) -> ("error out"=w1276:errorcluster)  [unwired: 7 in]
                }
                frame True {
                  n310 = Unbundle By Name(w1282) -> ("Calc.UCT.ALC"=w1287:sgl)
                  n311 = Greater Or Equal?(x=w1287, y=w1286) -> (x >= y?=w1285:bool)
                  n312 = case shown="True" w1285 {
                    tunnel: [RunTest_-_State."Idle" RunTest_-_State."Run"] -> w1290
                    tunnel: [w1301 w1304] -> w1289
                    tunnel: w1288 -> [w1300 w1304]
                    tunnel: w1287 -> [w1298 _]
                    tunnel: w1286 -> [w1297 _]
                    tunnel: w1284 -> [_ _]
                    tunnel: [w1294 w1307] -> w1283
                    tunnel: w1282 -> [w1293 w1306]
                    tunnel: w1281 -> [_ w1302]
                    frame False {
                      n313 = Unbundle By Name(w1293) -> ("Calc.UCT.Axial Strain"=w1292:sgl)
                      n314 = Format Into String(format string="Load Change %f < %f" ("Delay"), initial string="", error in=w1300, w1298, w1297) -> (resulting string=w1291:string, error out=w1301:errorcluster)
                      n315 = local write "Delay"(w1291) -> ()
                      n316 = Bundle By Name(cluster=w1293, "Log Prev Axial"=w1292) -> (w1294:T1)
                    }
                    frame True {
                      n317 = Bundle By Name(cluster=w1306, "Test RunTime"=w1302, "Stop.UCT.Prev Time"=w1302, "Calc.UCT.MaxDeviator"=sgl 0.0, "1st Log"=TRUE, "Log Prev Time"=w1302) -> (w1307:T1)
                    }
                  }
                }
              }
            }
            frame False {
              n318 = case shown="True" w1318 {
                tunnel: w1317 -> [w1323 w1329]
                tunnel: [w1323 w1329] -> w1315
                tunnel: w1316 -> [_ _]
                tunnel: w1314 -> [w1322 w1327]
                tunnel: [w1320 w1328] -> w1313
                tunnel: w1312 -> [_ _]
                tunnel: [RunTest_-_State."Idle" RunTest_-_State."Run"] -> w1311
                tunnel: w1310 -> [_ _]
                tunnel: w1309 -> [_ w1326]
                frame False {
                  n319 = Bundle By Name(cluster=w1322, "Start.UCT.PreStart"=TRUE ("Start.TS.PreStart")) -> (w1320:T1)
                }
                frame True {
                  n320 = Bundle By Name(cluster=w1327, "Test RunTime"=w1326, "Stop.UCT.Prev Time"=w1326, "Calc.UCT.MaxDeviator"=sgl 0.0, "1st Log"=TRUE, "Log Prev Time"=w1326) -> (w1328:T1)
                }
              }
            }
          }
        }
        frame True {
          n321 = case shown="False" w1333 {
            tunnel: [w1346 w1350] -> w1337
            tunnel: w1336 -> [w1345 w1350]
            tunnel: w1335 -> [w1344 _]
            tunnel: w1334 -> [w1340 _]
            tunnel: [w1343 w1351] -> w1332
            tunnel: w1331 -> [w1342 w1351]
            frame False {
              n322 = Bundle By Name(cluster=T12 {"Target Load"=0.0, "Target Disp"=0.0, "Rate"=0.0, "Speed"=0.0} ("Test"), "Speed"=w1340) -> (w1349:T12)
              n323 = Bundle By Name(cluster=w1342, "Start.UCT.Trig SS"=TRUE ("Start.TS.Trig SS")) -> (w1343:T1)
              n324 = call "Main - Set and Run PID (SubVI).vi"("Action"=T13."Run Disp", "error in (no error)"=w1345, "Test"=w1349, "IP Address"=w1344) -> ("error out"=w1346:errorcluster)  [unwired: 7 in]
            }
            frame True {
            }
          }
          n325 = case shown="True" w1338 {
            tunnel: [RunTest_-_State."Check Stop" RunTest_-_State."Check Post Stop"] -> w1339
            frame False {
            }
            frame True {
            }
          }
        }
      }
    }
    frame 9 {
      n326 = Unbundle By Name(w1358) -> ("Start.Iso.BP"=w1356:dbl, "Running?"=w1361:bool, "IP Address"=w1360:string[], "KeyName"=w1357:string[])
      n327 = case shown="False" w1361 {
        tunnel: [w1373 w1396] -> w1364
        tunnel: w1363 -> [w1382 w1395]
        tunnel: w1360 -> [w1381 w1392]
        tunnel: [RunTest_-_State."Run" RunTest_-_State."Check Stop"] -> w1362
        tunnel: [w1380 w1393] -> w1359
        tunnel: w1358 -> [w1371 w1393]
        tunnel: w1357 -> [w1378 w1391]
        tunnel: "BPC Iso" ("String") -> [w1379 w1390]
        tunnel: w1356 -> [w1370 w1394]
        tunnel: w1354 -> [w1366 _]
        frame False {
          n328 = Unbundle By Name(w1371) -> ("Sensor Data"=w1372:sgl[])
          n329 = Search 1D Array(1D array=w1378, element=w1379) -> (index of element=w1376:i32)  [unwired: 1 in]
          n330 = Index Array(array=w1372, index=2) -> (element=w1367:sgl)
          n331 = Index Array(array=w1381, index=w1376) -> (element=w1377:string)
          n332 = for {
            N: 3 -> [_]
            tunnel: w1377 -> [w1388]
            tunnel: w1370 -> [w1383]
            shift-right: [w1384] -> w1373
            shift-left: w1382 -> [w1389]
            n333 = Bundle By Name(cluster=T12 {"Target Load"=0.0, "Target Disp"=0.0, "Rate"=0.0, "Speed"=0.0} ("Test"), "Target Load"=w1383) -> (w1385:T12)
            n334 = call "Main - Set and Run PID (SubVI).vi"("Action"=T13."Run Target", "error in (no error)"=w1389, "Test"=w1385, "IP Address"=w1388) -> ("error out"=w1384:errorcluster)  [unwired: 7 in]
          }
          n335 = Unbundle By Name(w1371) -> ("Stop.Iso.Time2"=w1375:dbl)
          n336 = Add(x=w1375, y=w1366) -> (x+y=w1374:dbl)
          n337 = Bundle By Name(cluster=w1371, "Stop.Iso.Last Vc"=w1367, "Stop.Iso.Time Cond"=w1366, "Stop.Iso.Time Cond 2"=w1374, "Test RunTime"=w1366, "Log Prev Time"=w1366) -> (w1380:T1)
        }
        frame True {
          n338 = disable-structure shown="Enabled" {
            disable-tunnel: [w1405 w1423] -> w1396
            disable-tunnel: w1395 -> [w1404 w1423]
            disable-tunnel: w1394 -> [w1403 _]
            disable-tunnel: w1393 -> [w1402 _]
            disable-tunnel: w1392 -> [w1401 _]
            disable-tunnel: w1391 -> [w1400 _]
            disable-tunnel: w1390 -> [w1399 _]
            frame Disabled {
              n339 = Unbundle By Name(w1402) -> ("Sensor Data"=w1410:sgl[])
              n340 = Index Array(array=w1410, index=1) -> (element=w1407:sgl)
              n341 = Increment(x=w1403) -> (x+1=w1408:dbl)
              n342 = Decrement(x=w1403) -> (x-1=w1409:dbl)
              n343 = In Range and Coerce(upper limit=w1408, x=w1407, lower limit=w1409) -> (In Range?=w1398:bool)  [unwired: 1 out]
              n344 = case shown="False" w1398 {
                tunnel: [w1416 w1422] -> w1405
                tunnel: w1404 -> [w1415 w1422]
                tunnel: w1403 -> [w1414 _]
                tunnel: w1401 -> [w1413 _]
                tunnel: w1400 -> [w1412 _]
                tunnel: w1399 -> [w1411 _]
                frame False {
                  n345 = Search 1D Array(1D array=w1412, element=w1411) -> (index of element=w1420:i32)  [unwired: 1 in]
                  n346 = Bundle By Name(cluster=T12 {"Target Load"=0.0, "Target Disp"=0.0, "Rate"=0.0, "Speed"=0.0} ("Test"), "Target Load"=w1414) -> (w1417:T12)
                  n347 = Index Array(array=w1413, index=w1420) -> (element=w1421:string)
                  n348 = call "Main - Set and Run PID (SubVI).vi"("Action"=T13."Run Target", "error in (no error)"=w1415, "Test"=w1417, "IP Address"=w1421) -> ("error out"=w1416:errorcluster)  [unwired: 7 in]
                }
                frame True {
                }
              }
            }
            frame Enabled {
            }
          }
        }
      }
    }
    frame 10 {
      n349 = Unbundle By Name(w1425) -> ("Running?"=w1427:bool)
      n350 = case shown="True" w1427 {
        tunnel: [w1431 w1440] -> w1430
        tunnel: w1429 -> [w1431 w1440]
        tunnel: [RunTest_-_State."Run" RunTest_-_State."Check Stop"] -> w1428
        tunnel: [w1439 w1441] -> w1426
        tunnel: w1425 -> [w1437 w1441]
        tunnel: w1424 -> [w1434 _]
        frame False {
          n351 = Unbundle By Name(w1437) -> ("Stop.SP.Time"=w1438:dbl, "Stop.SP.MaxTime"=w1435:dbl)
          n352 = Add(x=w1438, y=w1434) -> (x+y=w1433:dbl)
          n353 = Add(x=w1435, y=w1434) -> (x+y=w1432:dbl)
          n354 = Bundle By Name(cluster=w1437, "Stop.SP.Time Cond"=w1433, "Stop.SP.Max Time Cond"=w1432, "Test RunTime"=w1434, "Log Prev Time"=w1434) -> (w1439:T1)
        }
        frame True {
        }
      }
    }
  }
  "Enum" <- w6
  "error out" <- w5
  "Cluster out" <- w3
